vi "main.vi"() -> ()   [LabVIEW 2019]
uses:
  <vilib>/vision/Image Controls.llb/IMAQ Image.ctl
  <vilib>/Utility/error.llb/DialogType.ctl
  <vilib>/measure/mamon.llb/Trigger Detection for 1 Channel.vi
  <vilib>/vision/NI_Vision_Development_Module.lvlib
  <vilib>/measure/NI_MAPro.lvlib
panel:
  out "Frame Rate":dbl
  out "Speed.ER":bool
  out "error out 7":errorcluster
  out "error out 6":errorcluster
  out "error out 5":errorcluster
  out "pallet Movement (m)":dbl format="%.2g"
  out "Plt Count 2":bool
  out "pallet count accept":bool
  out "machine pallet speed":dbl format="%#_3g"
  out "Array 2":errorcluster[](array[cluster])
  in  "Login":bool=TRUE
  out "error out 3":errorcluster
  out "GB sit 2":i8
  out "DEF TYPE":string="1"
  out "Sen.ER":bool
  out "Cam.ER":bool
  out "tcp read stop":bool
  out "main loop stop":bool
  out "event loop stop":bool
  out "sensor loop stop":bool
  out "stop ok":bool caption="YES"
  out "error out 2":errorcluster
  out "capture or not? 2":bool=TRUE
  out "stop live view":bool
  out "camera error out":errorcluster
  out "camera error in":errorcluster
  out "snap img":T1
  out "error out":errorcluster
  out "Array":dbl[][](array[numeric])
  out "SW&col sit":T2
  out "curv Array out":dbl[](array[numeric])
  out "capture or not?":bool=TRUE
  in  "Button":bool
  out "Frm False":bool
  out "Run/Stop":bool
  out "Sync":bool
  out "Speed (m/min) :":string="0"
  out "PLT NUM :":string="1"
  out "time&date 2":string="08:00:00"
  out "time&date":string="2020/11/22"
  out "Plt Count":bool
  out "Col. Count":bool
  in  "Sequence Button":bool
  in  "setting":bool
  in  "Graph Button":bool
  in  "report":bool
  in  "stop 3":bool
  out "DPIS":string="DPIS"
  in  "capture":bool
  out "Sen Plt\nNUM":i16
  out "CURV (mm)":dbl format="%#.2g"
  out "GB defects%":dbl format="%#.1g"
  out "Alarm":bool
  in  "OFF":bool
  out "Pallet Defects View":T1(plugin-control)
  out "GB sit":u32(colorbox)=16448250
  out "curv sit":bool
  out "SWR 2":bool
  out "SWL 2":bool
  in  "Refresh Button":bool
  in  "PLT NUM SYNC":i16
  out "Col\n NUM":dbl format="%#.1g"
  out "Live View":T1(plugin-control)
  out "bottum loop stop":bool
  out "stop ok":bool caption="OK"
  out "bottum refrence":refnum<vi>[](array[refnum])
  out "bottum array":bool[](array[boolean])
  in  "232":bool
  in  "231":bool
  in  "230":bool
  in  "229":bool
  in  "228":bool
  in  "227":bool
  in  "226":bool
  in  "225":bool
  in  "224":bool
  in  "223":bool
  in  "222":bool
  in  "221":bool
  in  "220":bool
  in  "219":bool
  in  "218":bool
  in  "217":bool
  in  "216":bool
  in  "215":bool
  in  "214":bool
  in  "213":bool
  in  "212":bool
  in  "211":bool
  in  "210":bool
  in  "209":bool
  in  "208":bool
  in  "207":bool
  in  "206":bool
  in  "205":bool
  in  "204":bool
  in  "203":bool
  in  "202":bool
  in  "201":bool
  in  "200":bool
  in  "199":bool
  in  "198":bool
  in  "197":bool
  in  "196":bool
  in  "195":bool
  in  "194":bool
  in  "193":bool
  in  "192":bool
  in  "191":bool
  in  "190":bool
  in  "189":bool
  in  "188":bool
  in  "187":bool
  in  "186":bool
  in  "185":bool
  in  "184":bool
  in  "183":bool
  in  "182":bool
  in  "181":bool
  in  "180":bool
  in  "179":bool
  in  "178":bool
  in  "177":bool
  in  "176":bool
  in  "175":bool
  in  "174":bool
  in  "173":bool
  in  "172":bool
  in  "171":bool
  in  "170":bool
  in  "169":bool
  in  "168":bool
  in  "167":bool
  in  "166":bool
  in  "165":bool
  in  "164":bool
  in  "163":bool
  in  "162":bool
  in  "161":bool
  in  "160":bool
  in  "159":bool
  in  "158":bool
  in  "157":bool
  in  "156":bool
  in  "155":bool
  in  "154":bool
  in  "153":bool
  in  "152":bool
  in  "151":bool
  in  "150":bool
  in  "149":bool
  in  "148":bool
  in  "147":bool
  in  "146":bool
  in  "145":bool
  in  "144":bool
  in  "143":bool
  in  "142":bool
  in  "141":bool
  in  "140":bool
  in  "139":bool
  in  "138":bool
  in  "137":bool
  in  "136":bool
  in  "135":bool
  in  "134":bool
  in  "133":bool
  in  "132":bool
  in  "131":bool
  in  "130":bool
  in  "129":bool
  in  "128":bool
  in  "127":bool
  in  "126":bool
  in  "125":bool
  in  "124":bool
  in  "123":bool
  in  "122":bool
  in  "121":bool
  in  "120":bool
  in  "119":bool
  in  "118":bool
  in  "117":bool
  in  "1":bool
  in  "2":bool
  in  "3":bool
  in  "4":bool
  in  "5":bool
  in  "6":bool
  in  "7":bool
  in  "8":bool
  in  "9":bool
  in  "10":bool
  in  "11":bool
  in  "12":bool
  in  "13":bool
  in  "14":bool
  in  "15":bool
  in  "16":bool
  in  "17":bool
  in  "18":bool
  in  "19":bool
  in  "20":bool
  in  "21":bool
  in  "22":bool
  in  "23":bool
  in  "24":bool
  in  "25":bool
  in  "26":bool
  in  "27":bool
  in  "28":bool
  in  "29":bool
  in  "30":bool
  in  "31":bool
  in  "32":bool
  in  "33":bool
  in  "34":bool
  in  "35":bool
  in  "36":bool
  in  "37":bool
  in  "38":bool
  in  "39":bool
  in  "40":bool
  in  "41":bool
  in  "42":bool
  in  "43":bool
  in  "44":bool
  in  "45":bool
  in  "46":bool
  in  "47":bool
  in  "48":bool
  in  "49":bool
  in  "50":bool
  in  "51":bool
  in  "52":bool
  in  "53":bool
  in  "54":bool
  in  "55":bool
  in  "56":bool
  in  "57":bool
  in  "58":bool
  in  "59":bool
  in  "60":bool
  in  "61":bool
  in  "62":bool
  in  "63":bool
  in  "64":bool
  in  "65":bool
  in  "66":bool
  in  "67":bool
  in  "68":bool
  in  "69":bool
  in  "70":bool
  in  "71":bool
  in  "72":bool
  in  "73":bool
  in  "74":bool
  in  "75":bool
  in  "76":bool
  in  "77":bool
  in  "78":bool
  in  "79":bool
  in  "80":bool
  in  "81":bool
  in  "82":bool
  in  "83":bool
  in  "84":bool
  in  "85":bool
  in  "86":bool
  in  "87":bool
  in  "88":bool
  in  "89":bool
  in  "90":bool
  in  "91":bool
  in  "92":bool
  in  "93":bool
  in  "94":bool
  in  "95":bool
  in  "96":bool
  in  "97":bool
  in  "98":bool
  in  "99":bool
  in  "100":bool
  in  "101":bool
  in  "102":bool
  in  "103":bool
  in  "104":bool
  in  "105":bool
  in  "106":bool
  in  "107":bool
  in  "108":bool
  in  "109":bool
  in  "110":bool
  in  "111":bool
  in  "112":bool
  in  "113":bool
  in  "114":bool
  in  "115":bool
  in  "116":bool
types:
  T1 = typedef "IMAQ Image.ctl" = refnum<image>
  T2 = cluster{"curv sit":bool, "Right Sidewall":bool, "Left SideWall":bool}
  T3 = typedef "Image Type" = u32
  T4 = enum8{"Enabled", "Disabled", "Disabled and Grayed Out"}
  T5 = typedef "DialogType.ctl" = u16
  T6 = cluster{"plt number dis":i16, "Table Name":string, "Database Name":string, "DB days to save":i16, "IP #":string, "Img Path":path, "Port":u16, "time out":u16, "madule path":path, "IP # speed":string, "counting device":enum16{"Sensors", "Line Speed", "Sensors&Speed"}}
  T7 = cluster{"ch sensor1":dbl, "ch sensor2":dbl, "chs ensor3":dbl, "ch sw sensor1":dbl, "ch sw sensor2":dbl}
  T8 = cluster{"low level read thr 1":dbl, "low level read thr 2":dbl, "low level read thr 3":dbl, "Debounce Time":dbl, "falling level thr":dbl, "counting role 2":enum16{"1st sensor", "2nd sensor", "3rd sensor", "1st+2nd", "1st+3rd", "2nd+3rd", "1st+2nd+3rd"}}
  T9 = enum16{"1st sensor", "2nd sensor", "3rd sensor", "1st+2nd", "1st+3rd", "2nd+3rd", "1st+2nd+3rd"}
  T10 = cluster{"Curv thr (mm)":dbl, "SW timout(s)":dbl, "SWR thr":dbl, "SWL thr ":dbl}
  T11 = cluster{"curv sit":bool, "right SideWall ":bool, "Left SideWall":bool}
  T12 = cluster{"min box size":dbl, "max box size":dbl, "box ratio":dbl, "min area size(gap)":dbl, "max area size (gap)":dbl, "min area (hole)":dbl, "max area (hole)":dbl}
  T13 = enum32{"Invalid", "Standard", "Closed", "Hidden", "Minimized", "Maximized"}
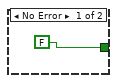
[diagram p3: hidden frame]
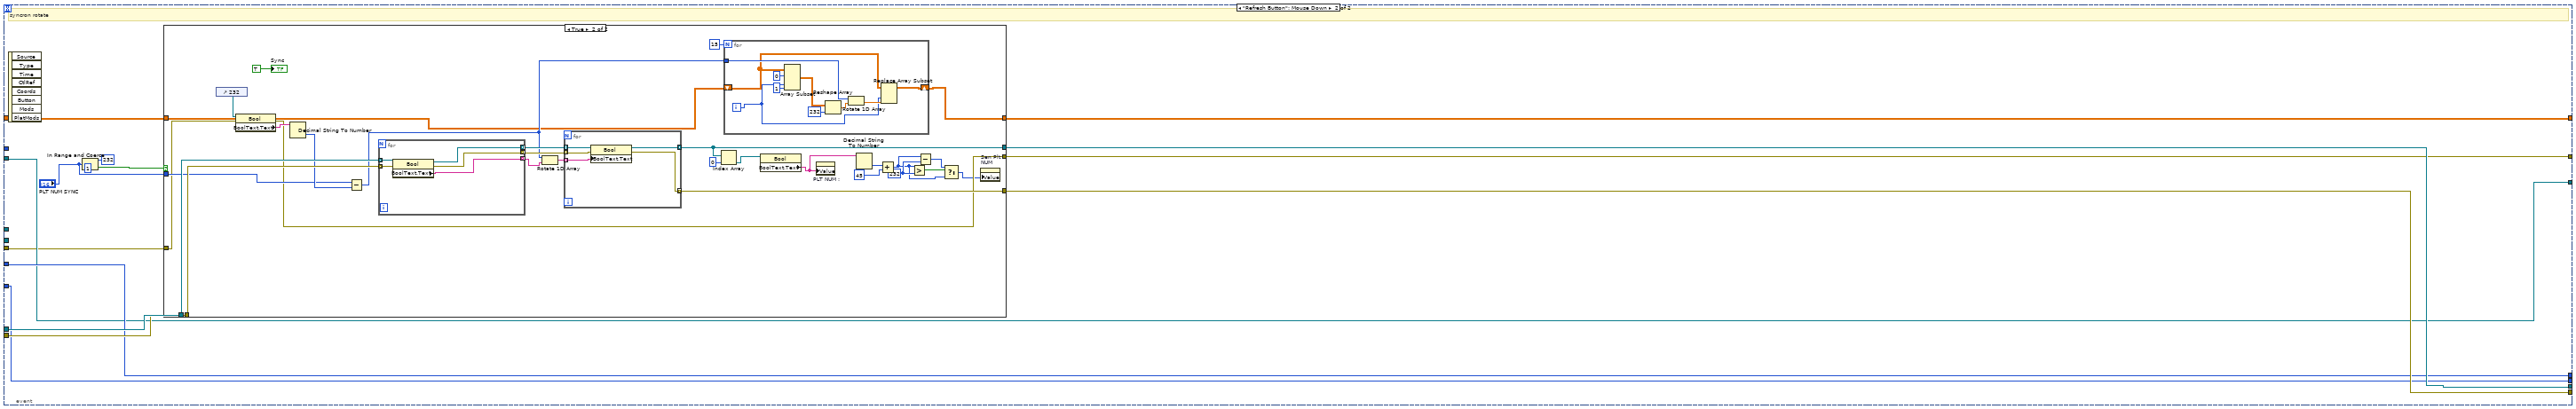
[diagram p6: hidden frame]
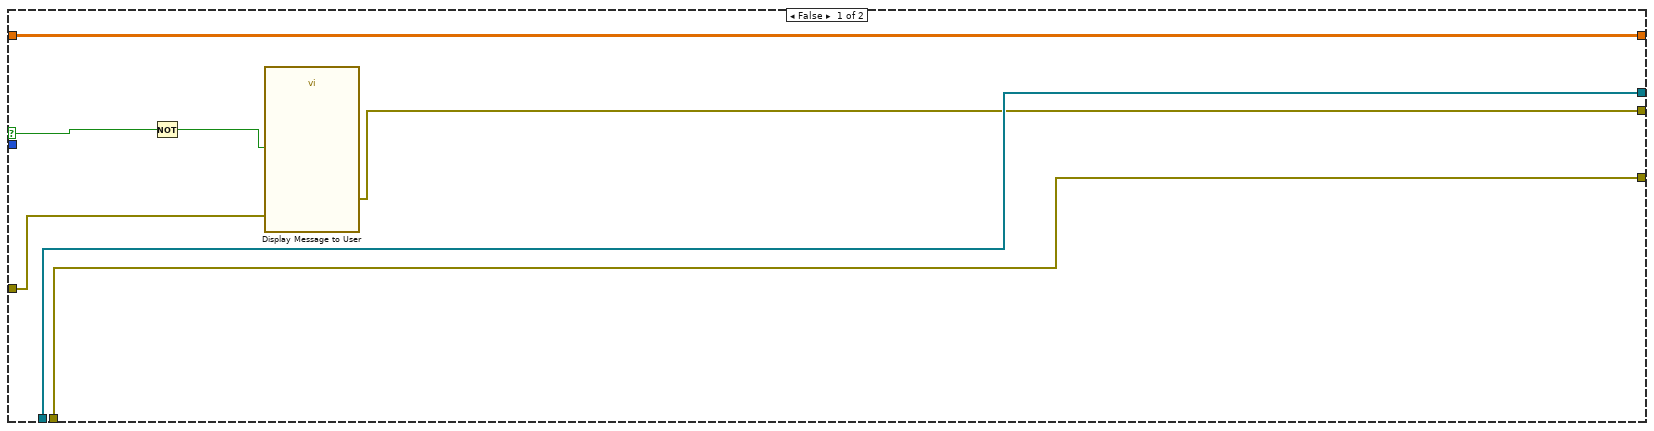
[diagram p7: hidden frame]
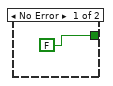
[diagram p8: hidden frame]
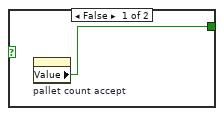
[diagram p10: hidden frame]
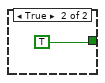
[diagram p11: hidden frame]
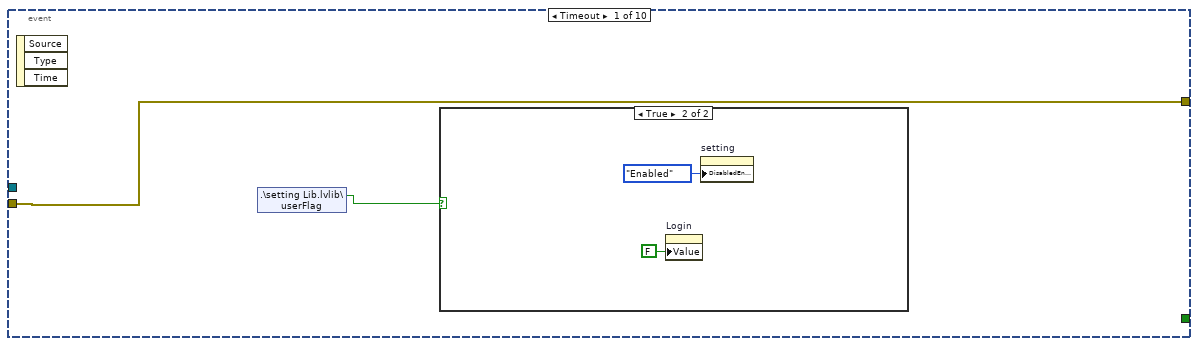
[diagram p12: hidden frame]
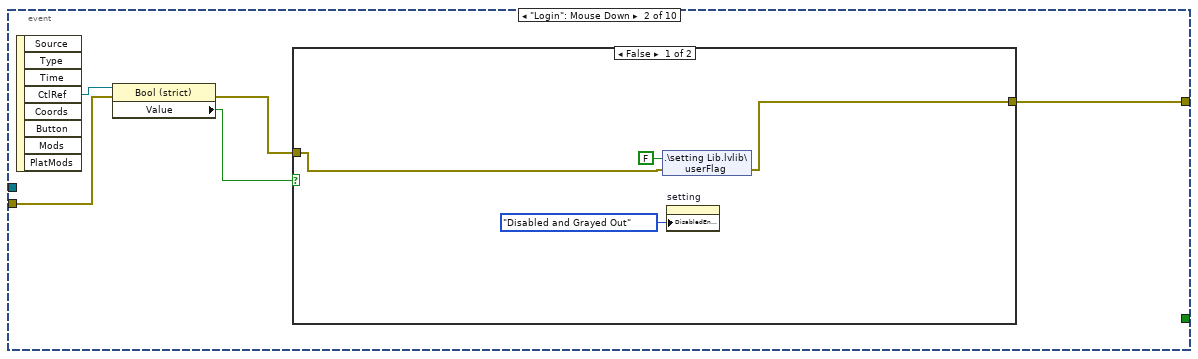
[diagram p14: hidden frame]
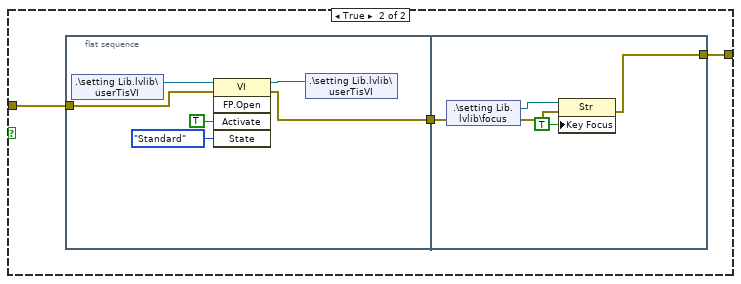
[diagram p15: hidden frame]
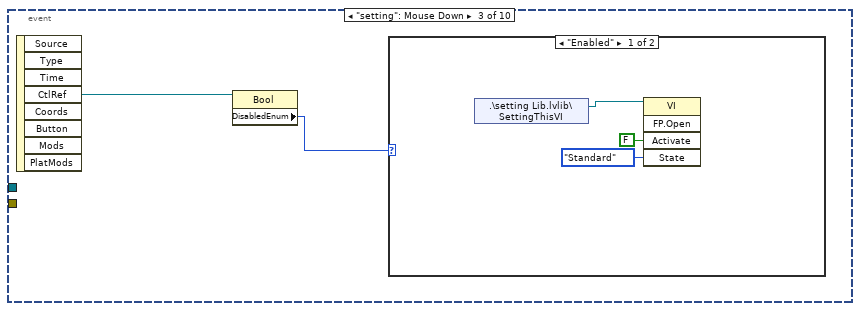
[diagram p16: hidden frame]
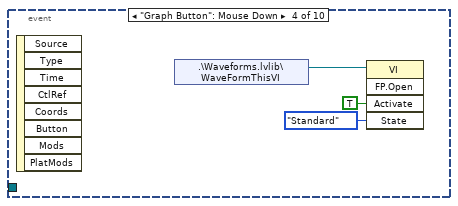
[diagram p18: hidden frame]
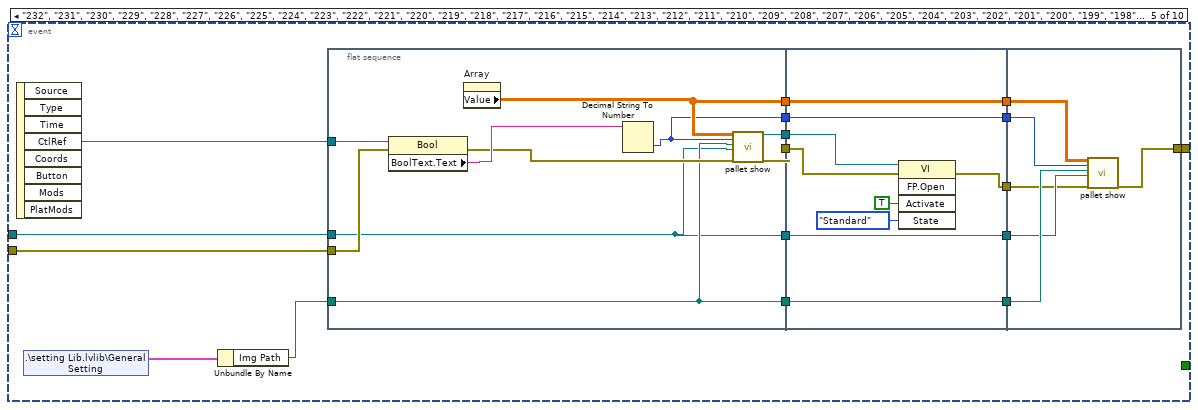
[diagram p19: hidden frame]
diagram:
  w2 = T3 0 items=["Grayscale (U8)", "Grayscale (I16)", "Grayscale (SGL)", "Complex (CSG)", "RGB (U32)", "HSL (U32)", "RGB (U64)", "Grayscale (U16)"] ("Image Type")
  w3 = T3 0 items=["Grayscale (U8)", "Grayscale (I16)", "Grayscale (SGL)", "Complex (CSG)", "RGB (U32)", "HSL (U32)", "RGB (U64)", "Grayscale (U16)"] ("Image Type")
  w32 = FALSE ("main loop stop")
  w40 = FALSE ("Plt Count")
  w59 = T3 4 items=["Grayscale (U8)", "Grayscale (I16)", "Grayscale (SGL)", "Complex (CSG)", "RGB (U32)", "HSL (U32)", "RGB (U64)", "Grayscale (U16)"] ("Image Type")
  w85 = 250 ("dimension size")
  w90 = 2 ("dimension size")
  w94 = 25 ("dimension size")
  n1 = while {
    tunnel: [w342] -> w109
    stop <- w342 stop-if-true
    n2 = Wait (ms)(milliseconds to wait=u32 5) -> ()  [unwired: 1 out]
    n3 = local read "stop ok"() -> (w342:bool)
    n4 = Build Array("232", "231", "230", "229", "228", "227", "226", "225", "224", "223", "222", "221", "220", "219", "218", "217", "216", "215", "214", "213", "212", "211", "210", "209", "208", "207", "206", "205", "204", "203", "202", "201", "200", "199", "198", "197", "196", "195", "194", "193", "192", "191", "190", "189", "188", "187", "186", "185", "184", "183", "182", "181", "180", "179", "178", "177", "176", "175", "174", "173", "172", "171", "170", "169", "168", "167", "166", "165", "164", "163", "162", "161", "160", "159", "158", "157", "156", "155", "154", "153", "152", "151", "150", "149", "148", "147", "146", "145", "144", "143", "142", "141", "140", "139", "138", "137", "136", "135", "134", "133", "132", "131", "130", "129", "128", "127", "126", "125", "124", "123", "122", "121", "120", "119", "118", "117", "116", "115", "114", "113", "112", "111", "110", "109", "108", "107", "106", "105", "104", "103", "102", "101", "100", "99", "98", "97", "96", "95", "94", "93", "92", "91", "90", "89", "88", "87", "86", "85", "84", "83", "82", "81", "80", "79", "78", "77", "76", "75", "74", "73", "72", "71", "70", "69", "68", "67", "66", "65", "64", "63", "62", "61", "60", "59", "58", "57", "56", "55", "54", "53", "52", "51", "50", "49", "48", "47", "46", "45", "44", "43", "42", "41", "40", "39", "38", "37", "36", "35", "34", "33", "32", "31", "30", "29", "28", "27", "26", "25", "24", "23", "22", "21", "20", "19", "18", "17", "16", "15", "14", "13", "12", "11", "10", "9", "8", "7", "6", "5", "4", "3", "2", "1") -> (→"bottum array":bool[])
  }
  "bottum loop stop" <- w109
  n5 = control-ref of="232"() -> (w341:refnum<vi>)
  n6 = control-ref of="231"() -> (w340:refnum<vi>)
  n7 = control-ref of="230"() -> (w339:refnum<vi>)
  n8 = control-ref of="229"() -> (w338:refnum<vi>)
  n9 = control-ref of="228"() -> (w337:refnum<vi>)
  n10 = control-ref of="227"() -> (w336:refnum<vi>)
  n11 = control-ref of="226"() -> (w335:refnum<vi>)
  n12 = control-ref of="225"() -> (w334:refnum<vi>)
  n13 = control-ref of="224"() -> (w333:refnum<vi>)
  n14 = control-ref of="223"() -> (w332:refnum<vi>)
  n15 = control-ref of="222"() -> (w331:refnum<vi>)
  n16 = control-ref of="221"() -> (w330:refnum<vi>)
  n17 = control-ref of="220"() -> (w329:refnum<vi>)
  n18 = control-ref of="219"() -> (w328:refnum<vi>)
  n19 = control-ref of="218"() -> (w327:refnum<vi>)
  n20 = control-ref of="217"() -> (w326:refnum<vi>)
  n21 = control-ref of="216"() -> (w325:refnum<vi>)
  n22 = control-ref of="215"() -> (w324:refnum<vi>)
  n23 = control-ref of="214"() -> (w323:refnum<vi>)
  n24 = control-ref of="213"() -> (w322:refnum<vi>)
  n25 = control-ref of="212"() -> (w321:refnum<vi>)
  n26 = control-ref of="211"() -> (w320:refnum<vi>)
  n27 = control-ref of="210"() -> (w319:refnum<vi>)
  n28 = control-ref of="209"() -> (w318:refnum<vi>)
  n29 = control-ref of="208"() -> (w317:refnum<vi>)
  n30 = control-ref of="207"() -> (w316:refnum<vi>)
  n31 = control-ref of="206"() -> (w315:refnum<vi>)
  n32 = control-ref of="205"() -> (w314:refnum<vi>)
  n33 = control-ref of="204"() -> (w313:refnum<vi>)
  n34 = control-ref of="203"() -> (w312:refnum<vi>)
  n35 = control-ref of="202"() -> (w311:refnum<vi>)
  n36 = control-ref of="201"() -> (w310:refnum<vi>)
  n37 = control-ref of="200"() -> (w309:refnum<vi>)
  n38 = control-ref of="199"() -> (w308:refnum<vi>)
  n39 = control-ref of="198"() -> (w307:refnum<vi>)
  n40 = control-ref of="197"() -> (w306:refnum<vi>)
  n41 = control-ref of="196"() -> (w305:refnum<vi>)
  n42 = control-ref of="195"() -> (w304:refnum<vi>)
  n43 = control-ref of="194"() -> (w303:refnum<vi>)
  n44 = control-ref of="193"() -> (w302:refnum<vi>)
  n45 = control-ref of="192"() -> (w301:refnum<vi>)
  n46 = control-ref of="191"() -> (w300:refnum<vi>)
  n47 = control-ref of="190"() -> (w299:refnum<vi>)
  n48 = control-ref of="189"() -> (w298:refnum<vi>)
  n49 = control-ref of="188"() -> (w297:refnum<vi>)
  n50 = control-ref of="187"() -> (w296:refnum<vi>)
  n51 = control-ref of="186"() -> (w295:refnum<vi>)
  n52 = control-ref of="185"() -> (w294:refnum<vi>)
  n53 = control-ref of="184"() -> (w293:refnum<vi>)
  n54 = control-ref of="183"() -> (w292:refnum<vi>)
  n55 = control-ref of="182"() -> (w291:refnum<vi>)
  n56 = control-ref of="181"() -> (w290:refnum<vi>)
  n57 = control-ref of="180"() -> (w289:refnum<vi>)
  n58 = control-ref of="179"() -> (w288:refnum<vi>)
  n59 = control-ref of="178"() -> (w287:refnum<vi>)
  n60 = control-ref of="177"() -> (w286:refnum<vi>)
  n61 = control-ref of="176"() -> (w285:refnum<vi>)
  n62 = control-ref of="175"() -> (w284:refnum<vi>)
  n63 = control-ref of="174"() -> (w283:refnum<vi>)
  n64 = control-ref of="173"() -> (w282:refnum<vi>)
  n65 = control-ref of="172"() -> (w281:refnum<vi>)
  n66 = control-ref of="171"() -> (w280:refnum<vi>)
  n67 = control-ref of="170"() -> (w279:refnum<vi>)
  n68 = control-ref of="169"() -> (w278:refnum<vi>)
  n69 = control-ref of="168"() -> (w277:refnum<vi>)
  n70 = control-ref of="167"() -> (w276:refnum<vi>)
  n71 = control-ref of="166"() -> (w275:refnum<vi>)
  n72 = control-ref of="165"() -> (w274:refnum<vi>)
  n73 = control-ref of="164"() -> (w273:refnum<vi>)
  n74 = control-ref of="163"() -> (w272:refnum<vi>)
  n75 = control-ref of="162"() -> (w271:refnum<vi>)
  n76 = control-ref of="161"() -> (w270:refnum<vi>)
  n77 = control-ref of="160"() -> (w269:refnum<vi>)
  n78 = control-ref of="159"() -> (w268:refnum<vi>)
  n79 = control-ref of="158"() -> (w267:refnum<vi>)
  n80 = control-ref of="157"() -> (w266:refnum<vi>)
  n81 = control-ref of="156"() -> (w265:refnum<vi>)
  n82 = control-ref of="155"() -> (w264:refnum<vi>)
  n83 = control-ref of="154"() -> (w263:refnum<vi>)
  n84 = control-ref of="153"() -> (w262:refnum<vi>)
  n85 = control-ref of="152"() -> (w261:refnum<vi>)
  n86 = control-ref of="151"() -> (w260:refnum<vi>)
  n87 = control-ref of="150"() -> (w259:refnum<vi>)
  n88 = control-ref of="149"() -> (w258:refnum<vi>)
  n89 = control-ref of="148"() -> (w257:refnum<vi>)
  n90 = control-ref of="147"() -> (w256:refnum<vi>)
  n91 = control-ref of="146"() -> (w255:refnum<vi>)
  n92 = control-ref of="145"() -> (w254:refnum<vi>)
  n93 = control-ref of="144"() -> (w253:refnum<vi>)
  n94 = control-ref of="143"() -> (w252:refnum<vi>)
  n95 = control-ref of="142"() -> (w251:refnum<vi>)
  n96 = control-ref of="141"() -> (w250:refnum<vi>)
  n97 = control-ref of="140"() -> (w249:refnum<vi>)
  n98 = control-ref of="139"() -> (w248:refnum<vi>)
  n99 = control-ref of="138"() -> (w247:refnum<vi>)
  n100 = control-ref of="137"() -> (w246:refnum<vi>)
  n101 = control-ref of="136"() -> (w245:refnum<vi>)
  n102 = control-ref of="135"() -> (w244:refnum<vi>)
  n103 = control-ref of="134"() -> (w243:refnum<vi>)
  n104 = control-ref of="133"() -> (w242:refnum<vi>)
  n105 = control-ref of="132"() -> (w241:refnum<vi>)
  n106 = control-ref of="131"() -> (w240:refnum<vi>)
  n107 = control-ref of="130"() -> (w239:refnum<vi>)
  n108 = control-ref of="129"() -> (w238:refnum<vi>)
  n109 = control-ref of="128"() -> (w237:refnum<vi>)
  n110 = control-ref of="127"() -> (w236:refnum<vi>)
  n111 = control-ref of="126"() -> (w235:refnum<vi>)
  n112 = control-ref of="125"() -> (w234:refnum<vi>)
  n113 = control-ref of="124"() -> (w233:refnum<vi>)
  n114 = control-ref of="123"() -> (w232:refnum<vi>)
  n115 = control-ref of="122"() -> (w231:refnum<vi>)
  n116 = control-ref of="121"() -> (w230:refnum<vi>)
  n117 = control-ref of="120"() -> (w229:refnum<vi>)
  n118 = control-ref of="119"() -> (w228:refnum<vi>)
  n119 = control-ref of="118"() -> (w227:refnum<vi>)
  n120 = control-ref of="117"() -> (w226:refnum<vi>)
  n121 = control-ref of="116"() -> (w225:refnum<vi>)
  n122 = control-ref of="115"() -> (w224:refnum<vi>)
  n123 = control-ref of="114"() -> (w223:refnum<vi>)
  n124 = control-ref of="113"() -> (w222:refnum<vi>)
  n125 = control-ref of="112"() -> (w221:refnum<vi>)
  n126 = control-ref of="111"() -> (w220:refnum<vi>)
  n127 = control-ref of="110"() -> (w219:refnum<vi>)
  n128 = control-ref of="109"() -> (w218:refnum<vi>)
  n129 = control-ref of="108"() -> (w217:refnum<vi>)
  n130 = control-ref of="107"() -> (w216:refnum<vi>)
  n131 = control-ref of="106"() -> (w215:refnum<vi>)
  n132 = control-ref of="105"() -> (w214:refnum<vi>)
  n133 = control-ref of="104"() -> (w213:refnum<vi>)
  n134 = control-ref of="103"() -> (w212:refnum<vi>)
  n135 = control-ref of="102"() -> (w211:refnum<vi>)
  n136 = control-ref of="101"() -> (w210:refnum<vi>)
  n137 = control-ref of="100"() -> (w209:refnum<vi>)
  n138 = control-ref of="99"() -> (w208:refnum<vi>)
  n139 = control-ref of="98"() -> (w207:refnum<vi>)
  n140 = control-ref of="97"() -> (w206:refnum<vi>)
  n141 = control-ref of="96"() -> (w205:refnum<vi>)
  n142 = control-ref of="95"() -> (w204:refnum<vi>)
  n143 = control-ref of="94"() -> (w203:refnum<vi>)
  n144 = control-ref of="93"() -> (w202:refnum<vi>)
  n145 = control-ref of="92"() -> (w201:refnum<vi>)
  n146 = control-ref of="91"() -> (w200:refnum<vi>)
  n147 = control-ref of="90"() -> (w199:refnum<vi>)
  n148 = control-ref of="89"() -> (w198:refnum<vi>)
  n149 = control-ref of="88"() -> (w197:refnum<vi>)
  n150 = control-ref of="87"() -> (w196:refnum<vi>)
  n151 = control-ref of="86"() -> (w195:refnum<vi>)
  n152 = control-ref of="85"() -> (w194:refnum<vi>)
  n153 = control-ref of="84"() -> (w193:refnum<vi>)
  n154 = control-ref of="83"() -> (w192:refnum<vi>)
  n155 = control-ref of="82"() -> (w191:refnum<vi>)
  n156 = control-ref of="81"() -> (w190:refnum<vi>)
  n157 = control-ref of="80"() -> (w189:refnum<vi>)
  n158 = control-ref of="79"() -> (w188:refnum<vi>)
  n159 = control-ref of="78"() -> (w187:refnum<vi>)
  n160 = control-ref of="77"() -> (w186:refnum<vi>)
  n161 = control-ref of="76"() -> (w185:refnum<vi>)
  n162 = control-ref of="75"() -> (w184:refnum<vi>)
  n163 = control-ref of="74"() -> (w183:refnum<vi>)
  n164 = control-ref of="73"() -> (w182:refnum<vi>)
  n165 = control-ref of="72"() -> (w181:refnum<vi>)
  n166 = control-ref of="71"() -> (w180:refnum<vi>)
  n167 = control-ref of="70"() -> (w179:refnum<vi>)
  n168 = control-ref of="69"() -> (w178:refnum<vi>)
  n169 = control-ref of="68"() -> (w177:refnum<vi>)
  n170 = control-ref of="67"() -> (w176:refnum<vi>)
  n171 = control-ref of="66"() -> (w175:refnum<vi>)
  n172 = control-ref of="65"() -> (w174:refnum<vi>)
  n173 = control-ref of="64"() -> (w173:refnum<vi>)
  n174 = control-ref of="63"() -> (w172:refnum<vi>)
  n175 = control-ref of="62"() -> (w171:refnum<vi>)
  n176 = control-ref of="61"() -> (w170:refnum<vi>)
  n177 = control-ref of="60"() -> (w169:refnum<vi>)
  n178 = control-ref of="59"() -> (w168:refnum<vi>)
  n179 = control-ref of="58"() -> (w167:refnum<vi>)
  n180 = control-ref of="57"() -> (w166:refnum<vi>)
  n181 = control-ref of="56"() -> (w165:refnum<vi>)
  n182 = control-ref of="55"() -> (w164:refnum<vi>)
  n183 = control-ref of="54"() -> (w163:refnum<vi>)
  n184 = control-ref of="53"() -> (w162:refnum<vi>)
  n185 = control-ref of="52"() -> (w161:refnum<vi>)
  n186 = control-ref of="51"() -> (w160:refnum<vi>)
  n187 = control-ref of="50"() -> (w159:refnum<vi>)
  n188 = control-ref of="49"() -> (w158:refnum<vi>)
  n189 = control-ref of="48"() -> (w157:refnum<vi>)
  n190 = control-ref of="47"() -> (w156:refnum<vi>)
  n191 = control-ref of="46"() -> (w155:refnum<vi>)
  n192 = control-ref of="45"() -> (w154:refnum<vi>)
  n193 = control-ref of="44"() -> (w153:refnum<vi>)
  n194 = control-ref of="43"() -> (w152:refnum<vi>)
  n195 = control-ref of="42"() -> (w151:refnum<vi>)
  n196 = control-ref of="41"() -> (w150:refnum<vi>)
  n197 = control-ref of="40"() -> (w149:refnum<vi>)
  n198 = control-ref of="39"() -> (w148:refnum<vi>)
  n199 = control-ref of="38"() -> (w147:refnum<vi>)
  n200 = control-ref of="37"() -> (w146:refnum<vi>)
  n201 = control-ref of="36"() -> (w145:refnum<vi>)
  n202 = control-ref of="35"() -> (w144:refnum<vi>)
  n203 = control-ref of="34"() -> (w143:refnum<vi>)
  n204 = control-ref of="33"() -> (w142:refnum<vi>)
  n205 = control-ref of="32"() -> (w141:refnum<vi>)
  n206 = control-ref of="31"() -> (w140:refnum<vi>)
  n207 = control-ref of="30"() -> (w139:refnum<vi>)
  n208 = control-ref of="29"() -> (w138:refnum<vi>)
  n209 = control-ref of="28"() -> (w137:refnum<vi>)
  n210 = control-ref of="27"() -> (w136:refnum<vi>)
  n211 = control-ref of="26"() -> (w135:refnum<vi>)
  n212 = control-ref of="25"() -> (w134:refnum<vi>)
  n213 = control-ref of="24"() -> (w133:refnum<vi>)
  n214 = control-ref of="23"() -> (w132:refnum<vi>)
  n215 = control-ref of="22"() -> (w131:refnum<vi>)
  n216 = control-ref of="21"() -> (w130:refnum<vi>)
  n217 = control-ref of="20"() -> (w129:refnum<vi>)
  n218 = control-ref of="19"() -> (w128:refnum<vi>)
  n219 = control-ref of="18"() -> (w127:refnum<vi>)
  n220 = control-ref of="17"() -> (w126:refnum<vi>)
  n221 = control-ref of="16"() -> (w125:refnum<vi>)
  n222 = control-ref of="15"() -> (w124:refnum<vi>)
  n223 = control-ref of="14"() -> (w123:refnum<vi>)
  n224 = control-ref of="13"() -> (w122:refnum<vi>)
  n225 = control-ref of="12"() -> (w121:refnum<vi>)
  n226 = control-ref of="11"() -> (w120:refnum<vi>)
  n227 = control-ref of="10"() -> (w119:refnum<vi>)
  n228 = control-ref of="9"() -> (w118:refnum<vi>)
  n229 = control-ref of="8"() -> (w117:refnum<vi>)
  n230 = control-ref of="7"() -> (w116:refnum<vi>)
  n231 = control-ref of="6"() -> (w115:refnum<vi>)
  n232 = control-ref of="5"() -> (w114:refnum<vi>)
  n233 = control-ref of="4"() -> (w113:refnum<vi>)
  n234 = control-ref of="3"() -> (w112:refnum<vi>)
  n235 = control-ref of="2"() -> (w111:refnum<vi>)
  n236 = control-ref of="1"() -> (w110:refnum<vi>)
  n237 = property on="Run/Stop" class="Bool (strict)"("Blinking"=FALSE) -> ()  [unwired: 2 in, 2 out]
  n238 = property on="Alarm" class="Bool (strict)"("Blinking"=FALSE) -> ()  [unwired: 2 in, 2 out]
  n239 = property on="Sync" class="Bool (strict)"("Value"=FALSE ("Sync")) -> ()  [unwired: 2 in, 2 out]
  n240 = property on="Run/Stop" class="Bool (strict)"("Value"=TRUE ("Run/Stop")) -> ()  [unwired: 2 in, 2 out]
  n241 = property on="event loop stop" class="Bool (strict)"("Value"=w32) -> ()  [unwired: 2 in, 2 out]
  n242 = property on="tcp read stop" class="Bool (strict)"("Value"=w32) -> ()  [unwired: 2 in, 2 out]
  n243 = property on="stop live view" class="Bool (strict)"("Value"=w32) -> ()  [unwired: 2 in, 2 out]
  n244 = property on="sensor loop stop" class="Bool (strict)"("Value"=w32) -> ()  [unwired: 2 in, 2 out]
  n245 = property on="main loop stop" class="Bool (strict)"("Value"=w32) -> ()  [unwired: 2 in, 2 out]
  n246 = property on="Col\n NUM" class="DigNum (strict)"("Value"=0.0 ("Col\n NUM")) -> ()  [unwired: 2 in, 2 out]
  n247 = property on="Sen Plt\nNUM" class="DigNum (strict)"("Value"=i16 46 ("Sen Plt\nNUM")) -> ()  [unwired: 2 in, 2 out]
  n248 = property on="PLT NUM SYNC" class="DigNum (strict)"("Value"=i16 1 ("PLT NUM SYNC")) -> ()  [unwired: 2 in, 2 out]
  n249 = property on="CURV (mm)" class="DigNum (strict)"("Value"=0.0 ("CURV (mm)")) -> ()  [unwired: 2 in, 2 out]
  n250 = property on="GB defects%" class="DigNum (strict)"("Value"=0.0 ("GB defects%")) -> ()  [unwired: 2 in, 2 out]
  n251 = property on="PLT NUM :" class="Str"("Value"="1" ("PLT NUM :")) -> ()  [unwired: 2 in, 2 out]
  n252 = Build Array(w341, w340, w339, w338, w337, w336, w335, w334, w333, w332, w331, w330, w329, w328, w327, w326, w325, w324, w323, w322, w321, w320, w319, w318, w317, w316, w315, w314, w313, w312, w311, w310, w309, w308, w307, w306, w305, w304, w303, w302, w301, w300, w299, w298, w297, w296, w295, w294, w293, w292, w291, w290, w289, w288, w287, w286, w285, w284, w283, w282, w281, w280, w279, w278, w277, w276, w275, w274, w273, w272, w271, w270, w269, w268, w267, w266, w265, w264, w263, w262, w261, w260, w259, w258, w257, w256, w255, w254, w253, w252, w251, w250, w249, w248, w247, w246, w245, w244, w243, w242, w241, w240, w239, w238, w237, w236, w235, w234, w233, w232, w231, w230, w229, w228, w227, w226, w225, w224, w223, w222, w221, w220, w219, w218, w217, w216, w215, w214, w213, w212, w211, w210, w209, w208, w207, w206, w205, w204, w203, w202, w201, w200, w199, w198, w197, w196, w195, w194, w193, w192, w191, w190, w189, w188, w187, w186, w185, w184, w183, w182, w181, w180, w179, w178, w177, w176, w175, w174, w173, w172, w171, w170, w169, w168, w167, w166, w165, w164, w163, w162, w161, w160, w159, w158, w157, w156, w155, w154, w153, w152, w151, w150, w149, w148, w147, w146, w145, w144, w143, w142, w141, w140, w139, w138, w137, w136, w135, w134, w133, w132, w131, w130, w129, w128, w127, w126, w125, w124, w123, w122, w121, w120, w119, w118, w117, w116, w115, w114, w113, w112, w111, w110) -> (w108:refnum<vi>[])
  "bottum refrence" <- w108
  n253 = while {
    tunnel: errorcluster {"status"=FALSE, "code"=0, "source"=""} ("error in (no error)") -> [w589]
    tunnel: [w585] -> w99
    tunnel: [w584] -> w98
    tunnel: [w577] -> w33
    stop <- w577 stop-if-true
    w586 = T5 0 items=["no dialog", "OK message", "continue or stop message", "OK message + warnings", "continue/stop + warnings"] ("type of dialog (OK msg:1)")
    n254 = shared-variable ".\\setting Lib.lvlib\\General Setting"() -> (w583:T6)  [unwired: 1 in, 1 out]
    n255 = Unbundle By Name(w583) -> ("IP #"=w582:string, "Port"=w581:u16)
    n256 = TCP Open Connection(address=w582, remote port or service name=w581, timeout ms (60000)=-1, error in (no error)=w589) -> (connection ID=w585:refnum<k5>, error out=w588:errorcluster)  [unwired: 1 in]
    n257 = shared-variable ".\\setting Lib.lvlib\\StopOk"() -> (w579:bool)  [unwired: 1 in, 1 out]
    n258 = call <vilib>:"Simple Error Handler.vi"("type of dialog (OK msg:1)"=w586, "error in (no error)"=w588) -> ("error?"=w587:bool, "error out"=w584:errorcluster)  [unwired: 3 in, 3 out]
    n259 = Not(x=w587) -> (.not. x?=w578:bool)
    n260 = Wait (ms)(milliseconds to wait=u32 5) -> ()  [unwired: 1 out]
    n261 = Or(x=w579, y=w578) -> (x .or. y?=w577:bool)
  }
  "tcp read stop" <- w33
  n262 = while {
    tunnel: errorcluster {"status"=FALSE, "code"=0, "source"=""} ("error in (no error)") -> [w603]
    tunnel: [w599] -> w19
    tunnel: [w598] -> w18
    tunnel: [w592] -> _
    stop <- w592 stop-if-true
    w600 = T5 0 items=["no dialog", "OK message", "continue or stop message", "OK message + warnings", "continue/stop + warnings"] ("type of dialog (OK msg:1)")
    n263 = shared-variable ".\\setting Lib.lvlib\\General Setting"() -> (w597:T6)  [unwired: 1 in, 1 out]
    n264 = Unbundle By Name(w597) -> ("IP # speed"=w596:string, "Port"=w591:u16)
    n265 = TCP Open Connection(address=w596, remote port or service name=w591, timeout ms (60000)=-1, error in (no error)=w603) -> (connection ID=w599:refnum<k5>, error out=w602:errorcluster)  [unwired: 1 in]
    n266 = shared-variable ".\\setting Lib.lvlib\\StopOk"() -> (w594:bool)  [unwired: 1 in, 1 out]
    n267 = call <vilib>:"Simple Error Handler.vi"("type of dialog (OK msg:1)"=w600, "error in (no error)"=w602) -> ("error?"=w601:bool, "error out"=w598:errorcluster)  [unwired: 3 in, 3 out]
    n268 = Not(x=w601) -> (.not. x?=w593:bool)
    n269 = Wait (ms)(milliseconds to wait=u32 5) -> ()  [unwired: 1 out]
    n270 = Or(x=w594, y=w593) -> (x .or. y?=w592:bool)
  }
  n271 = call "IMAQ Create"("Image Name"="mainimg", "Image Type"=w3, "error in (no error)"=errorcluster {"status"=FALSE, "code"=0, "source"=""}) -> ("New Image"=w56:T1, "error out"=w4:errorcluster)  [unwired: 2 in]
  n272 = control-ref of="Button"() -> (w107:refnum<vi>)
  n273 = property class="Bool"(reference=w107) -> ("Colors [4]"=w106:cluster{u32, u32}[])  [unwired: 1 in, 2 out]
  n274 = Initialize Array(i16 0 ("element"), 232 ("dimension size")) -> (w103:i16[])
  n275 = call "IMAQ Create"("Image Name"="rotate", "Image Type"=w2, "error in (no error)"=w4) -> ("New Image"=w49:T1, "error out"=w1:errorcluster)  [unwired: 2 in]
  n276 = for {
    tunnel: w108 -> [w617] mode=indexing
    tunnel: w106 -> [w612]
    shift-right: [w607] -> _
    shift-left: w103 -> [w609]
    tunnel: [w606] -> w102 mode=indexing
    tunnel: [w605] -> w101 mode=indexing
    i -> [w608]
    # "initialize text and label and colour of pallets"
    n277 = property class="Bool"(reference=w617) -> (reference out=w616:refnum<vi>, error out=w614:errorcluster, "Label.Text"=w615:string)  [unwired: 1 in]
    n278 = Replace Array Subset(array=w609, new element=w608, index=w608) -> (w607:i16[])
    n279 = property class="Bool"(reference=w616, error in=w614, "BoolText.Text"=w615) -> (reference out=w613:refnum<vi>)  [unwired: 1 out]
    n280 = property class="Bool"(reference=w613, "Colors [4]"=w612) -> (reference out=w611:refnum<vi>)  [unwired: 1 in, 1 out]
    n281 = property class="Bool"(reference=w611, "DisabledEnum"=T4."Disabled and Grayed Out" ("Disabled")) -> (reference out=w606:refnum<vi>, error out=w605:errorcluster)  [unwired: 1 in]
  }
  n282 = property on="capture or not?" class="Bool (strict)"("Value"=FALSE ("capture")) -> ()  [unwired: 2 in, 2 out]
  n283 = Open Python Session(python version="3.6" ("Python version"), 3:errorcluster {"status"=FALSE, "code"=0, "source"=""} ("error in (no error)")) -> (session out=w77:refnum<k35>, error out=w43:errorcluster)  [unwired: 1 in]
  n284 = while {
    tunnel: w56 -> [w638]
    tunnel: [w626] -> w53
    tunnel: [w630] -> w51
    tunnel: w49 -> [w639]
    tunnel: [w622] -> w48
    tunnel: w1 -> [w618]
    stop <- w626 stop-if-true
    # "Live view"
    n285 = flat-sequence {
      tunnel: w638 -> [w642]
      tunnel: w639 -> [w643]
      tunnel: [w643] -> w621
      tunnel: [w642] -> w620
      tunnel: [w641] -> w619
      tunnel: w618 -> [w641]
      tunnel: [w646] -> w637
      tunnel: [w644] -> w636
      tunnel: [w648] -> w635
      tunnel: [w647] -> w634
      tunnel: w621 -> [w648]
      tunnel: w620 -> [w647]
      tunnel: w619 -> [_]
      tunnel: w637 -> [w649]
      tunnel: w636 -> [w651]
      tunnel: w635 -> [w655]
      tunnel: w634 -> [w652]
      tunnel: [w655] -> w633
      tunnel: [w654] -> w632
      tunnel: [w650] -> w631
      tunnel: [w650] -> w627
      tunnel: w633 -> [w658]
      tunnel: w632 -> [w660]
      tunnel: w631 -> [w659]
      tunnel: [w661] -> w629
      tunnel: [w657] -> w628
      tunnel: w627 -> [w656]
      tunnel: [w662] -> w630
      tunnel: [w663] -> w622
      tunnel: w628 -> [w662]
      tunnel: w629 -> [w663]
      frame #0 {
      }
      frame #1 {
        (unwired) 10000 ("Timeout (ms)")
        n286 = call "Vision Acquisition"() -> ("Image Out"=w644:T1, "Frame Rate"=→"Frame Rate":dbl, "error out"=w646:errorcluster)  [unwired: 24 in, 1 out]
      }
      frame #2 {
        n287 = call "IMAQ Rotate"("error in (no error)"=w649, "Angle (degrees)"=sgl 180.0, "Image Dst"=w652, "Image Src"=w651) -> ("error out"=w654:errorcluster, "Image Dst Out"=w650:T1)  [unwired: 6 in]
      }
      frame #3 {
        n288 = call "IMAQ Copy"("error in (no error)"=w660, "Image Dst"=w658, "Image Src"=w659) -> ("error out"=w661:errorcluster, "Image Dst Out"=w657:T1)  [unwired: 3 in]
        "Live View" <- w656
      }
      frame #4 {
        "snap img" <- w662
      }
    }
    n289 = Wait (ms)(milliseconds to wait=u32 20) -> ()  [unwired: 1 out]
    n290 = shared-variable ".\\setting Lib.lvlib\\StopOk"() -> (w626:bool)  [unwired: 1 in, 1 out]
    n291 = Select(t=TRUE, s=w622, f=FALSE) -> (s? t:f=→"Cam.ER":bool)
    "camera error in" <- w622
  }
  "stop live view" <- w53
  n292 = Initialize Array(0.0 ("element"), w90, 2 ("dimension size")) -> (w91:dbl[][])
  n293 = Initialize Array(0.0 ("element"), w94, 3 ("dimension size")) -> (w95:dbl[][])
  n294 = property on="Col. Count" class="Bool (strict)"("Value"=FALSE ("Col. Count")) -> ()  [unwired: 2 in, 2 out]
  n295 = shared-variable ".\\setting Lib.lvlib\\StopOk"(FALSE ("StopOk")) -> ()  [unwired: 1 in, 1 out]
  n296 = call "IMAQ Create"("Image Name"="img crop", "error in (no error)"=w43) -> ("New Image"=w73:T1, "error out"=w74:errorcluster)  [unwired: 3 in]
  n297 = Initialize Array(0.0 ("element"), 6 ("dimension size")) -> (w81:dbl[])
  n298 = Initialize Array(0.0 ("element"), w85, 3 ("dimension size")) -> (w86:dbl[][])
  n299 = while {
    tunnel: w19 -> [w681]
    tunnel: w18 -> [w680]
    tunnel: [w669] -> w13
    stop <- FALSE stop-if-true
    n300 = call "adamread.vi"("TCP Connection Refnum in"=w681, "error in (no error)"=w680) -> ("Slave Input Registers 2"=w679:dbl[], "error out 2"=w669:errorcluster)  [unwired: 11 in, 1 out]
    n301 = Index Array(array=w679, index=3) -> (element=w677:dbl)
    n302 = Multiply(x=w677, y=0.000129) -> (x*y=w665:dbl)
    n303 = Greater?(x=w665, y=3.5) -> (0:w667:bool)
    n304 = case shown="False" w667 {
      tunnel: w665 -> [w683 w685]
      tunnel: [w684 w685] -> w664
      frame False {
        n305 = Multiply(x=w683, y=1.04) -> (x*y=w684:dbl)
      }
      frame True {
      }
    }
    "machine pallet speed" <- w664
    n306 = Number To Fractional String(number=w664, precision (6)=i16 2 ("width (-)")) -> (F-format string=→"Speed (m/min) :":string)  [unwired: 2 in]
    n307 = Greater?(x=w664, y=0.5) -> (0:→"Run/Stop":bool)
    n308 = case shown="Error .." w669 {
      tunnel: [FALSE ("Speed.ER") TRUE ("Speed.ER")] -> w668
      frame No Error {
      }
      frame Error {
      }
    }
    "Speed.ER" <- w668
    n309 = Wait (ms)(milliseconds to wait=u32 2000) -> ()  [unwired: 1 out]
  }
  "error out 7" <- w13
  n310 = Initialize Array(u32 0 ("element"), 400 ("dimension size"), 4 ("dimension size")) -> (w67:u32[][])
  n311 = Initialize Array "Crv&Sw info"(0.0 ("element"), 232 ("dimension size"), 16 ("dimension size")) -> (w63:dbl[][])
  n312 = call "IMAQ Create"("Image Name"="img out", "error in (no error)"=w74) -> ("New Image"=w72:T1, "error out"=w75:errorcluster)  [unwired: 3 in]
  n313 = call "defects database show.vi"() -> ()  [unwired: 12 in]
  n314 = call "query 2.vi"() -> ()  [unwired: 27 in, 1 out]
  n315 = Initialize Array(0.0 ("element"), 2 ("dimension size")) -> (w6:dbl[])
  n316 = Initialize Array(0.0 ("element"), 2 ("dimension size")) -> (w15:dbl[])
  n317 = property on="setting" class="Bool"("DisabledEnum"=T4."Disabled and Grayed Out" ("Disabled")) -> ()  [unwired: 2 in, 2 out]
  n318 = property on="capture or not? 2" class="Bool (strict)"("Value"=FALSE ("capture or not? 2")) -> ()  [unwired: 2 in, 2 out]
  n319 = call "user login.vi"() -> ()  [unwired: 12 in]
  n320 = property on="Plt Count" class="Bool (strict)"("Value"=w40) -> ()  [unwired: 2 in, 2 out]
  n321 = property on="Col. Count" class="Bool (strict)"("Value"=w40) -> ()  [unwired: 2 in, 2 out]
  n322 = call "setting page 2.vi"() -> ()  [unwired: 15 in, 1 out]
  n323 = call "IMAQ Create"("Image Name"="pallet show", "Image Type"=w59, "error in (no error)"=errorcluster {"status"=FALSE, "code"=0, "source"=""}) -> ("New Image"=w60:T1, "error out"=w42:errorcluster)  [unwired: 2 in]
  n324 = shared-variable ".\\setting Lib.lvlib\\userFlag"(FALSE ("userFlag")) -> ()  [unwired: 1 in, 1 out]
  n325 = property on="Login" class="Bool (strict)"("Value"=TRUE ("Login")) -> ()  [unwired: 2 in, 2 out]
  n326 = while {
    tunnel: w99 -> [w800]
    tunnel: w98 -> [w799]
    tunnel: w94 -> [w797]
    tunnel: w90 -> [w795]
    shift-right: [w792] -> _
    shift-left: w95 -> [w798]
    shift-right: [w791] -> _
    shift-left: w91 -> [w796]
    shift-right: [w773] -> _
    shift-left: i8 0 -> [w794]
    tunnel: w85 -> [w780]
    shift-right: [w777] -> _
    shift-left: w86 -> [w784]
    shift-right: [w768] -> _
    shift-left: w81 -> [w771]
    tunnel: [w726] -> w38
    tunnel: [w725] -> w37
    tunnel: [w724] -> w36
    shift-right: [w714] -> _
    shift-left: w15 -> [w715]
    shift-right: [w696] -> _
    shift-left: w6 -> [w699]
    stop <- w724 stop-if-true
    # "Sensors reading"
    n327 = shared-variable ".\\setting Lib.lvlib\\ChannelSetting"() -> (w723:T7)  [unwired: 1 in, 1 out]
    n328 = property on="capture or not? 2" class="Bool (strict)"() -> ("Value"=w688:bool)  [unwired: 2 in, 2 out]
    n329 = flat-sequence {
      tunnel: w800 -> [w843]
      tunnel: w799 -> [w842]
      tunnel: [w841] -> w815
      tunnel: w798 -> [w841]
      tunnel: [w840] -> w814
      tunnel: w797 -> [w840]
      tunnel: [w839] -> w813
      tunnel: w796 -> [w839]
      tunnel: [w838] -> w812
      tunnel: w795 -> [w838]
      tunnel: [w837] -> w811
      tunnel: w794 -> [w837]
      tunnel: [w836] -> w785
      tunnel: w784 -> [w836]
      tunnel: [w835] -> w781
      tunnel: w780 -> [w835]
      tunnel: [w834] -> w772
      tunnel: w771 -> [w834]
      tunnel: [w827] -> w751
      tunnel: [w818] -> w738
      tunnel: [w826] -> w727
      tunnel: w723 -> [w825]
      tunnel: [w817] -> w722
      tunnel: [w819] -> w716
      tunnel: w715 -> [w819]
      tunnel: w699 -> [w816]
      tunnel: [w816] -> w697
      tunnel: w815 -> [w872]
      tunnel: w814 -> [w871]
      tunnel: w813 -> [w870]
      tunnel: w812 -> [w869]
      tunnel: [w868] -> w810
      tunnel: [w867] -> w809
      tunnel: [w847] -> w808
      tunnel: [w866] -> w807
      tunnel: w811 -> [w866]
      tunnel: [w865] -> w806
      tunnel: [w864] -> w786
      tunnel: w785 -> [w864]
      tunnel: [w863] -> w782
      tunnel: w781 -> [w863]
      tunnel: w772 -> [w862]
      tunnel: [w862] -> w769
      tunnel: [w861] -> w758
      tunnel: [w860] -> w757
      tunnel: [w859] -> w756
      tunnel: [w848] -> w755
      tunnel: [w858] -> w754
      tunnel: [w857] -> w753
      tunnel: [w856] -> w752
      tunnel: w751 -> [w849]
      tunnel: w738 -> [w854]
      tunnel: [w853] -> w737
      tunnel: [w852] -> w728
      tunnel: w727 -> [w852]
      tunnel: w722 -> [w851]
      tunnel: [w850] -> w717
      tunnel: w716 -> [w850]
      tunnel: [w847] -> w702
      tunnel: [w846] -> w698
      tunnel: w697 -> [w846]
      tunnel: w810 -> [w901]
      tunnel: w809 -> [w900]
      tunnel: w808 -> [w885]
      tunnel: w807 -> [w884]
      tunnel: w806 -> [w899]
      tunnel: [w901] -> w805
      tunnel: [w900] -> w804
      tunnel: [w885] -> w803
      tunnel: [w899] -> w802
      tunnel: [w882] -> w801
      tunnel: [w898] -> w787
      tunnel: w786 -> [w898]
      tunnel: [w897] -> w783
      tunnel: w782 -> [w897]
      tunnel: [w892] -> w779
      tunnel: [w878] -> w778
      tunnel: [w896] -> w770
      tunnel: w769 -> [w896]
      tunnel: w758 -> [w895]
      tunnel: w757 -> [w894]
      tunnel: w756 -> [w893]
      tunnel: w755 -> [w880]
      tunnel: w754 -> [w876]
      tunnel: w753 -> [w883]
      tunnel: w752 -> [w887]
      tunnel: [w873] -> w744
      tunnel: [w888] -> w743
      tunnel: [w875] -> w739
      tunnel: w737 -> [w891]
      tunnel: [w874] -> w736
      tunnel: [w890] -> w729
      tunnel: w728 -> [w890]
      tunnel: [w889] -> w718
      tunnel: w717 -> [w889]
      tunnel: w702 -> [w888]
      tunnel: w698 -> [w879]
      tunnel: [w881] -> w691
      tunnel: w688 -> [w873]
      tunnel: w805 -> [w921]
      tunnel: w804 -> [w920]
      tunnel: w803 -> [w914]
      tunnel: w802 -> [w913]
      tunnel: w801 -> [w911]
      tunnel: [w921] -> w790
      tunnel: [w920] -> w789
      tunnel: [w911] -> w788
      tunnel: w787 -> [w919]
      tunnel: w783 -> [w918]
      tunnel: w779 -> [w917]
      tunnel: w778 -> [w916]
      tunnel: [w915] -> w776
      tunnel: [w914] -> w775
      tunnel: [w913] -> w774
      tunnel: w770 -> [w912]
      tunnel: [w910] -> w767
      tunnel: [w910] -> w766
      tunnel: [w909] -> w745
      tunnel: w744 -> [w909]
      tunnel: w743 -> [w908]
      tunnel: [w907] -> w740
      tunnel: w739 -> [w907]
      tunnel: w736 -> [w906]
      tunnel: [w905] -> w735
      tunnel: [w904] -> w730
      tunnel: w729 -> [w904]
      tunnel: [w903] -> w719
      tunnel: w718 -> [w903]
      tunnel: [w902] -> w692
      tunnel: w691 -> [w902]
      tunnel: w790 -> [w939]
      tunnel: w789 -> [w938]
      tunnel: w788 -> [w929]
      tunnel: w776 -> [w937]
      tunnel: w775 -> [w936]
      tunnel: w774 -> [w932]
      tunnel: w767 -> [w935]
      tunnel: w766 -> [w933]
      tunnel: [w939] -> w765
      tunnel: [w938] -> w764
      tunnel: [w930] -> w763
      tunnel: [w937] -> w762
      tunnel: [w935] -> w761
      tunnel: [w933] -> w760
      tunnel: [w932] -> w759
      tunnel: w745 -> [w922]
      tunnel: [w928] -> w741
      tunnel: w740 -> [w928]
      tunnel: w735 -> [w927]
      tunnel: [w926] -> w734
      tunnel: [w925] -> w731
      tunnel: w730 -> [w925]
      tunnel: [w924] -> w720
      tunnel: w719 -> [w924]
      tunnel: [w923] -> w693
      tunnel: w692 -> [w923]
      tunnel: [w922] -> w690
      tunnel: w765 -> [w965]
      tunnel: w764 -> [w964]
      tunnel: w763 -> [w957]
      tunnel: w762 -> [w963]
      tunnel: w761 -> [w962]
      tunnel: w760 -> [w961]
      tunnel: w759 -> [w958]
      tunnel: [w965] -> w750
      tunnel: [w964] -> w749
      tunnel: [w957] -> w748
      tunnel: [w963] -> w747
      tunnel: [w962] -> w746
      tunnel: [w951] -> w742
      tunnel: w741 -> [w951]
      tunnel: w734 -> [w950]
      tunnel: [w944] -> w733
      tunnel: [w949] -> w732
      tunnel: w731 -> [w949]
      tunnel: [w945] -> w721
      tunnel: w720 -> [w945]
      tunnel: [w942] -> w694
      tunnel: w693 -> [w942]
      tunnel: w690 -> [w940]
      tunnel: [w940] -> w689
      tunnel: w732 -> [w980]
      tunnel: w733 -> [w974]
      tunnel: w742 -> [w977]
      tunnel: w750 -> [w985]
      tunnel: w749 -> [w984]
      tunnel: w748 -> [w983]
      tunnel: w747 -> [w982]
      tunnel: w746 -> [w981]
      tunnel: w721 -> [w979]
      tunnel: [w985] -> w713
      tunnel: [w984] -> w712
      tunnel: [w983] -> w711
      tunnel: [w982] -> w710
      tunnel: [w981] -> w709
      tunnel: [w973] -> w708
      tunnel: [w980] -> w707
      tunnel: [w978] -> w706
      tunnel: [w975] -> w705
      tunnel: [w975] -> w704
      tunnel: [w976] -> w701
      tunnel: [w975] -> w700
      tunnel: [w972] -> w695
      tunnel: w694 -> [w972]
      tunnel: w689 -> [w967]
      tunnel: [w996] -> w714
      tunnel: [w997] -> w726
      tunnel: [w987] -> w725
      tunnel: [w998] -> w768
      tunnel: [w999] -> w777
      tunnel: [w1000] -> w773
      tunnel: [w1001] -> w791
      tunnel: [w1002] -> w792
      tunnel: w713 -> [w1002]
      tunnel: w712 -> [w1001]
      tunnel: w711 -> [w1000]
      tunnel: w710 -> [w999]
      tunnel: w709 -> [w998]
      tunnel: w708 -> [w988]
      tunnel: w707 -> [w997]
      tunnel: w706 -> [w996]
      tunnel: w705 -> [w995]
      tunnel: w704 -> [w994]
      tunnel: [w993] -> w703
      tunnel: w701 -> [w989]
      tunnel: w700 -> [_]
      tunnel: [w986] -> w696
      tunnel: w695 -> [w986]
      frame #0 {
        # "sensor data read"
        n330 = Unbundle By Name(w825) -> ("ch sensor1"=w824:dbl, "ch sensor2"=w823:dbl, "chs ensor3"=w822:dbl, "ch sw sensor1"=w821:dbl, "ch sw sensor2"=w820:dbl)
        n331 = call "adamread.vi"("TCP Connection Refnum in"=w843, "error in (no error)"=w842) -> ("TCP Connection Refnum (dup)"=w826:refnum<k5>, "Slave Input Registers 2"=w833:dbl[], "error out 2"=w818:errorcluster)  [unwired: 11 in]
        n332 = case shown="Error .." w818 {
          tunnel: [FALSE ("error?") TRUE ("error?")] -> w817
          frame No Error {
          }
          frame Error {
          }
        }
        n333 = Index Array(array=w833, index #1=w824, index #2=w823, index #3=w822, index #4=w821, index #5=w820) -> (element #1=w832:dbl, element #2=w831:dbl, element #3=w830:dbl, element #4=w829:dbl, element #5=w828:dbl)
        n334 = Build Array(w832, w831, w830, w829, w828) -> (w827:dbl[])
      }
      frame #1 {
        # "Averaging of sesor pallet"
        n335 = shared-variable ".\\setting Lib.lvlib\\CurvSetting"(error in=w854) -> (w855:T8, error out=w853:errorcluster)
        n336 = shared-variable ".\\setting Lib.lvlib\\RisingSensorThr"() -> (w856:dbl[])  [unwired: 1 in, 1 out]
        n337 = call "Waveform Averaging.vi"("2D curv array in"=w872, "array sensor in"=w849, "avg wind1"=w871, "2D Sw Array In"=w870, "avg Win2"=w869) -> ("2D curv Array out"=w868:dbl[][], "2D Sw Array Out"=w867:dbl[][], "Curv Average Array Out"=w847:dbl[], "SW Average Array Out"=w865:dbl[])  [unwired: 11 in]
        n338 = property on="machine pallet speed" class="DigNum (strict)"() -> ("Value"=w848:dbl)  [unwired: 2 in, 2 out]
        n339 = Unbundle By Name(w855) -> ("low level read thr 1"=w861:dbl, "low level read thr 2"=w860:dbl, "low level read thr 3"=w859:dbl, "falling level thr"=w858:dbl, "counting role 2"=w857:T9)  [unwired: 1 out]
        "Sen.ER" <- w851
      }
      frame #2 {
        # "count coloumns and pallet"
        n340 = Build Array(w895, w894, w893) -> (w892:dbl[])
        n341 = property on="capture or not?" class="Bool (strict)"(error in=w891) -> (error out=w877:errorcluster, "Value"=w886:bool)  [unwired: 1 in, 1 out]
        n342 = call "sensor count.vi"("sensor thr array"=w887, "pallet speed"=w880, "speed array in"=w879, "capture y or no ?"=w886, "sensor data"=w885, "counter input"=w884, "counting role"=w883, "error in"=w877, "falling level thr"=w876) -> ("column count"=w878:bool, "speed array out"=w881:dbl[], "counter out"=w882:i8, "pallet detect"=w875:bool, "error out"=w874:errorcluster)  [unwired: 2 out]
        "Col. Count" <- w878
      }
      frame #3 {
        # "Curv Measuement"
        n343 = call "curvness detection.vi"("2D curv array in"=w919, "array sensor in"=w908, "avg wind1"=w918, "min level thr"=w917, "coloumn count"=w916, "curv Array"=w912, "col count"=w911, "error in (no error)"=w906) -> ("2D curv array Out"=w915:dbl[][], "curv Array out"=w910:dbl[], "error out"=w905:errorcluster)  [unwired: 8 in, 1 out]
      }
      frame #4 {
        # "Trends Show"
        n344 = property on="Sen Plt\nNUM" class="DigNum (strict)"(error in=w927) -> (error out=w926:errorcluster, "Value"=w934:i16)  [unwired: 1 in, 1 out]
        n345 = Select(t=i8 0, s=w922, f=w929) -> (s? t:f=w930:i8)
        "Col\n NUM" <- w930
        n346 = call "waveform show.vi"("curv array in"=w936, "SW array in"=w932, "Col Count 2"=w929, "coloumn curvness array"=w933, "Sensor Pallet NUM 2"=w934) -> ()  [unwired: 15 in]
      }
      frame #5 {
        # "SideWall and Curvensee situation set \nSideWall and Curvness situation set"
        n347 = shared-variable ".\\setting Lib.lvlib\\SW&CurvSetting"(error in=w950) -> (w955:T10, error out=w941:errorcluster)
        n348 = Index Array(array=w961, index=5) -> (element=w959:dbl)
        "CURV (mm)" <- w959
        n349 = property on="GB sit 2" class="DigNum (strict)"() -> ("Value"=w948:i8)  [unwired: 2 in, 2 out]
        n350 = call "sW&col situation.vi"("Overal CURV(mm)"=w959, "SW array in"=w958, "curv and Sw setting"=w955, "col count"=w957, "capture"=w940, "error in (no error)"=w941) -> ("curv sit"=w954:bool, "right SideWall"=w953:bool, "Left SideWall"=w952:bool, "error out"=w944:errorcluster)  [unwired: 9 in, 1 out]
        "curv sit" <- w954
        "SWL 2" <- w952
        "SWR 2" <- w953
        n351 = Equal?(x=w948, y=i8 2) -> (x = y?=w946:bool)
        n352 = Bundle("curv sit"=w954, "right SideWall"=w953, "Left SideWall"=w952) -> (→"SW&col sit":T11)  [unwired: 1 in]
        n353 = Compound Arithmetic op=OR(w954, w953, w952, w946) -> (w943:bool)
        n354 = case shown="True" w943 {
          tunnel: w943 -> [_ _]
          frame False {
          }
          frame True {
            w966 = TRUE
            n355 = property on="Alarm" class="Bool (strict)"("Blinking"=w966) -> ()  [unwired: 2 in, 2 out]
            n356 = property on="Alarm" class="Bool (strict)"("Value"=w966) -> ()  [unwired: 2 in, 2 out]
          }
        }
        "curv Array out" <- w961
      }
      frame #6 {
        n357 = property on="capture or not?" class="Bool (strict)"() -> ("Value"=w971:bool)  [unwired: 2 in, 2 out]
        n358 = property on="machine pallet speed" class="DigNum (strict)"() -> ("Value"=w970:dbl)  [unwired: 2 in, 2 out]
        n359 = call "speed&col syncroun 2.vi"("speed array in"=w979, "speed"=w970, "width"=1.6, "start"=w971, "instant capture"=w967, "acceptable width"=1.2, "plt count"=w977, "error in (no error)"=w974) -> ("total movement"=w976:dbl, "speed array out"=w978:dbl[], "plt count accept"=w975:bool, "error out"=w973:errorcluster)  [unwired: 6 in, 2 out]
        "Plt Count" <- w977
      }
      frame #7 {
        n360 = call "Elapsed Time"("Reset"=w995, "error in (no error)"=w988) -> ("Elapsed Time (s)"=w992:dbl, "error out"=w987:errorcluster)  [unwired: 10 in, 6 out]
        n361 = Greater Or Equal?(x=w992, y=1.0) -> (x >= y?=w990:bool)
        n362 = case shown="False" w994 {
          tunnel: [w1003 TRUE] -> w993
          tunnel: w990 -> [w1004 _]
          frame False {
            n363 = case shown="True" w1004 {
              tunnel: [w1005 FALSE ("Value")] -> w1003
              frame False {
                n364 = property on="pallet count accept" class="Bool (strict)"() -> ("Value"=w1005:bool)  [unwired: 2 in, 2 out]
              }
              frame True {
              }
            }
          }
          frame True {
          }
        }
        "pallet Movement (m)" <- w989
      }
    }
    n365 = Wait (ms)(milliseconds to wait=u32 10) -> ()  [unwired: 1 out]
    n366 = shared-variable ".\\setting Lib.lvlib\\StopOk"() -> (w724:bool)  [unwired: 1 in, 1 out]
    "pallet count accept" <- w703
    "Plt Count 2" <- w703
    "error out 6" <- w725
  }
  "sensor loop stop" <- w36
  n367 = while {
    shift-right: [w1024] -> _
    shift-left: 0 -> [w1025]
    shift-right: [w1023] -> _
    shift-left: w102 -> [w1027]
    shift-right: [w1016] -> _
    shift-left: 0 -> [w1021]
    tunnel: w77 -> [w1019]
    tunnel: w73 -> [w1018]
    tunnel: w72 -> [w1017]
    tunnel: [w1015] -> w71
    tunnel: w67 -> [w1014]
    shift-right: [w1010] -> _
    shift-left: w63 -> [w1013]
    tunnel: w75 -> [w1020]
    tunnel: [w1009] -> w58
    tunnel: w101 -> [w1026]
    tunnel: [w1022] -> w21
    tunnel: [w1008] -> w34
    stop <- w1008 stop-if-true
    # "Main Loop"
    n368 = event shown="[0] Timeout" {
      selector: _ -> [_ _]
      dyn-events: _ -> [_ _]
      timeout: 0 -> [_ _]
      tunnel: w1027 -> [w1059 w1536]
      tunnel: w1026 -> [w1058 w1535]
      tunnel: w1025 -> [w1057 w1531]
      tunnel: [w1056 w1531] -> w1024
      tunnel: [w1055 w1534] -> w1023
      tunnel: [w1054 w1533] -> w1022
      tunnel: w1021 -> [w1052 w1532]
      tunnel: w1020 -> [w1051 w1524]
      tunnel: w1019 -> [w1050 w1530]
      tunnel: w1018 -> [w1049 _]
      tunnel: w1017 -> [w1048 _]
      tunnel: [w1047 w1532] -> w1016
      tunnel: [w1046 w1530] -> w1015
      tunnel: w1014 -> [w1045 _]
      tunnel: w1013 -> [w1044 w1529]
      tunnel: [w1043 w1528] -> w1010
      tunnel: [w1035 w1523] -> w1009
      event Timeout {
        w1029 = u16 1 items=["Falling Edge", "Rising Edge"] ("trigger slope")
        n369 = event-data() -> ()  [unwired: 1 in, 3 out]
        n370 = shared-variable ".\\setting Lib.lvlib\\General Setting"() -> (w1038:T6)  [unwired: 1 in, 1 out]
        n371 = Get Date/Time In Seconds() -> (seconds since 1Jan1904=w1042:timestamp)
        n372 = property on="pallet count accept" class="Bool (strict)"() -> ("Value"=w1031:bool)  [unwired: 2 in, 2 out]
        n373 = Boolean To (0,1)(Boolean=w1031) -> (0, 1=w1032:i16)
        n374 = property on="capture or not? 2" class="Bool (strict)"() -> ("Value"=w1028:bool)  [unwired: 2 in, 2 out]
        n375 = Get Date/Time String(seconds (now)=w1042, want seconds? (F)=TRUE) -> (date string=→"time&date 2":string, time string=→"time&date":string)  [unwired: 1 in]
        n376 = Build Array(w1032) -> (w1033:i16[])
        n377 = call-poly <vilib>:"Basic Level Trigger Detection.vi"("signal in"=w1033, "level"=0.5, "trigger slope"=w1029) -> ("trigger detected?"=w1030:bool)  [unwired: 10 in, 2 out]
        n378 = Unbundle By Name(w1038) -> ("madule path"=w1037:path, "Img Path"=w1036:path)
        n379 = Or(x=w1030, y=w1028) -> (x .or. y?=w1053:bool)
        n380 = case shown="True" w1053 {
          tunnel: w1059 -> [w1065 w1204]
          tunnel: w1058 -> [w1064 w1203]
          tunnel: [w1065 w1202] -> w1055
          tunnel: [w1064 w1201] -> w1054
          tunnel: w1057 -> [w1066 w1200]
          tunnel: [w1066 w1199] -> w1056
          tunnel: w1052 -> [w1063 w1198]
          tunnel: w1051 -> [w1060 w1195]
          tunnel: w1050 -> [w1062 w1186]
          tunnel: w1049 -> [_ w1183]
          tunnel: w1048 -> [_ w1181]
          tunnel: [w1063 w1175] -> w1047
          tunnel: [w1062 w1172] -> w1046
          tunnel: w1045 -> [_ w1171]
          tunnel: w1044 -> [w1061 w1167]
          tunnel: [w1061 w1122] -> w1043
          tunnel: w1037 -> [_ w1097]
          tunnel: w1036 -> [_ w1095]
          tunnel: [w1060 w1076] -> w1035
          frame False {
          }
          frame True {
            n381 = flat-sequence {
              tunnel: w1200 -> [w1220]
              tunnel: w1203 -> [w1221]
              tunnel: w1204 -> [w1222]
              tunnel: [w1222] -> w1210
              tunnel: [w1221] -> w1209
              tunnel: [w1220] -> w1208
              tunnel: w1198 -> [w1219]
              tunnel: [w1218] -> w1197
              tunnel: w1195 -> [w1217]
              tunnel: [w1217] -> w1193
              tunnel: [w1216] -> w1187
              tunnel: w1186 -> [w1216]
              tunnel: [w1215] -> w1184
              tunnel: w1183 -> [w1215]
              tunnel: [w1214] -> w1182
              tunnel: w1181 -> [w1214]
              tunnel: w1171 -> [w1213]
              tunnel: [w1213] -> w1168
              tunnel: [w1212] -> w1098
              tunnel: w1097 -> [w1212]
              tunnel: [w1211] -> w1096
              tunnel: w1095 -> [w1211]
              tunnel: [w1240] -> w1207
              tunnel: [w1237] -> w1206
              tunnel: [w1236] -> w1205
              tunnel: w1210 -> [w1248]
              tunnel: w1209 -> [w1254]
              tunnel: w1208 -> [w1241]
              tunnel: w1197 -> [w1232]
              tunnel: [w1231] -> w1196
              tunnel: [w1230] -> w1194
              tunnel: w1193 -> [w1230]
              tunnel: [w1229] -> w1188
              tunnel: w1187 -> [w1229]
              tunnel: w1184 -> [w1228]
              tunnel: w1182 -> [w1227]
              tunnel: [w1228] -> w1179
              tunnel: [w1227] -> w1177
              tunnel: [w1226] -> w1173
              tunnel: [w1225] -> w1169
              tunnel: w1168 -> [w1225]
              tunnel: [w1224] -> w1100
              tunnel: w1098 -> [w1224]
              tunnel: w1096 -> [w1223]
              tunnel: [w1223] -> w1093
              tunnel: w1207 -> [w1300]
              tunnel: w1206 -> [w1299]
              tunnel: w1205 -> [w1298]
              tunnel: w1196 -> [_]
              tunnel: w1194 -> [w1291]
              tunnel: [w1300] -> w1192
              tunnel: [w1299] -> w1191
              tunnel: [w1298] -> w1190
              tunnel: [w1297] -> w1189
              tunnel: w1188 -> [w1297]
              tunnel: [w1287] -> w1185
              tunnel: [w1296] -> w1180
              tunnel: w1179 -> [w1296]
              tunnel: [w1295] -> w1178
              tunnel: w1177 -> [w1295]
              tunnel: [w1292] -> w1176
              tunnel: [w1294] -> w1174
              tunnel: w1173 -> [w1294]
              tunnel: [w1293] -> w1170
              tunnel: w1169 -> [w1293]
              tunnel: [w1290] -> w1101
              tunnel: w1100 -> [w1289]
              tunnel: [w1289] -> w1099
              tunnel: [w1288] -> w1094
              tunnel: w1093 -> [w1288]
              tunnel: [w1324] -> w1166
              tunnel: [w1323] -> w1165
              tunnel: [w1322] -> w1164
              tunnel: [w1321] -> w1163
              tunnel: [w1320] -> w1162
              tunnel: [w1319] -> w1161
              tunnel: [w1318] -> w1160
              tunnel: [w1305] -> w1159
              tunnel: w1170 -> [_]
              tunnel: w1174 -> [w1321]
              tunnel: w1176 -> [w1313]
              tunnel: w1178 -> [w1314]
              tunnel: w1180 -> [w1315]
              tunnel: w1185 -> [w1316]
              tunnel: w1189 -> [w1317]
              tunnel: w1190 -> [w1322]
              tunnel: w1191 -> [w1323]
              tunnel: w1192 -> [w1324]
              tunnel: [w1312] -> w1148
              tunnel: w1101 -> [w1311]
              tunnel: w1099 -> [w1309]
              tunnel: w1094 -> [w1308]
              tunnel: [w1308] -> w1091
              tunnel: [w1307] -> w1087
              tunnel: w1166 -> [w1346]
              tunnel: w1165 -> [w1345]
              tunnel: w1164 -> [w1344]
              tunnel: w1163 -> [w1343]
              tunnel: w1162 -> [w1342]
              tunnel: w1161 -> [w1340]
              tunnel: [w1346] -> w1158
              tunnel: [w1345] -> w1157
              tunnel: [w1344] -> w1156
              tunnel: [w1343] -> w1155
              tunnel: [w1342] -> w1154
              tunnel: [w1338] -> w1153
              tunnel: [w1337] -> w1152
              tunnel: w1160 -> [w1337]
              tunnel: [w1336] -> w1151
              tunnel: w1159 -> [w1336]
              tunnel: [w1335] -> w1150
              tunnel: [w1334] -> w1149
              tunnel: w1148 -> [w1334]
              tunnel: [w1333] -> w1147
              tunnel: [w1327] -> w1114
              tunnel: [w1326] -> w1092
              tunnel: w1091 -> [w1326]
              tunnel: [w1325] -> w1088
              tunnel: w1087 -> [w1325]
              tunnel: w1158 -> [w1375]
              tunnel: [w1375] -> w1146
              tunnel: w1157 -> [w1374]
              tunnel: [w1374] -> w1144
              tunnel: w1156 -> [w1373]
              tunnel: [w1373] -> w1142
              tunnel: w1155 -> [w1372]
              tunnel: [w1372] -> w1140
              tunnel: w1154 -> [w1371]
              tunnel: [w1371] -> w1138
              tunnel: w1153 -> [w1370]
              tunnel: [w1370] -> w1136
              tunnel: [w1355] -> w1134
              tunnel: w1152 -> [w1369]
              tunnel: [w1369] -> w1132
              tunnel: w1151 -> [w1368]
              tunnel: [w1368] -> w1130
              tunnel: w1150 -> [w1347]
              tunnel: w1149 -> [w1363]
              tunnel: w1147 -> [w1362]
              tunnel: [w1361] -> w1124
              tunnel: w1114 -> [w1359]
              tunnel: [w1351] -> w1103
              tunnel: [w1350] -> w1102
              tunnel: w1092 -> [w1349]
              tunnel: [w1348] -> w1089
              tunnel: w1088 -> [w1348]
              tunnel: w1146 -> [w1397]
              tunnel: [w1397] -> w1145
              tunnel: w1144 -> [w1396]
              tunnel: [w1396] -> w1143
              tunnel: w1142 -> [w1395]
              tunnel: [w1395] -> w1141
              tunnel: w1140 -> [w1394]
              tunnel: [w1394] -> w1139
              tunnel: w1138 -> [w1393]
              tunnel: [w1393] -> w1137
              tunnel: w1136 -> [w1392]
              tunnel: [w1392] -> w1135
              tunnel: w1134 -> [w1391]
              tunnel: [w1391] -> w1133
              tunnel: w1132 -> [w1390]
              tunnel: [w1390] -> w1131
              tunnel: w1130 -> [w1389]
              tunnel: [w1389] -> w1129
              tunnel: [w1388] -> w1128
              tunnel: [w1383] -> w1127
              tunnel: [w1382] -> w1126
              tunnel: [w1381] -> w1125
              tunnel: w1124 -> [w1380]
              tunnel: [w1379] -> w1123
              tunnel: w1103 -> [w1378]
              tunnel: w1102 -> [w1377]
              tunnel: [w1376] -> w1090
              tunnel: w1089 -> [w1376]
              tunnel: w1145 -> [w1449]
              tunnel: w1143 -> [w1448]
              tunnel: w1141 -> [w1447]
              tunnel: w1139 -> [w1446]
              tunnel: w1137 -> [w1445]
              tunnel: w1135 -> [w1404]
              tunnel: w1167 -> [w1444]
              tunnel: w1133 -> [w1407]
              tunnel: w1131 -> [w1430]
              tunnel: w1129 -> [w1429]
              tunnel: w1128 -> [w1428]
              tunnel: w1127 -> [w1414]
              tunnel: w1126 -> [w1413]
              tunnel: w1125 -> [w1412]
              tunnel: w1123 -> [w1411]
              tunnel: [w1449] -> w1121
              tunnel: [w1448] -> w1120
              tunnel: [w1447] -> w1119
              tunnel: [w1446] -> w1118
              tunnel: [w1445] -> w1117
              tunnel: [w1410] -> w1116
              tunnel: [w1409] -> w1115
              tunnel: [w1404] -> w1113
              tunnel: [w1407] -> w1112
              tunnel: w1090 -> [w1399]
              tunnel: w1121 -> [w1480]
              tunnel: w1120 -> [w1484]
              tunnel: w1119 -> [w1483]
              tunnel: w1118 -> [w1482]
              tunnel: w1117 -> [w1481]
              tunnel: w1116 -> [w1476]
              tunnel: w1115 -> [w1455]
              tunnel: w1113 -> [w1451]
              tunnel: w1112 -> [w1450]
              tunnel: [w1480] -> w1111
              tunnel: [w1484] -> w1110
              tunnel: [w1483] -> w1109
              tunnel: [w1482] -> w1108
              tunnel: [w1481] -> w1107
              tunnel: [w1454] -> w1106
              tunnel: [w1462] -> w1105
              tunnel: [w1461] -> w1104
              tunnel: [w1451] -> w1079
              tunnel: [w1450] -> w1078
              tunnel: w1111 -> [w1501]
              tunnel: w1110 -> [w1500]
              tunnel: w1109 -> [w1499]
              tunnel: w1108 -> [w1498]
              tunnel: w1107 -> [w1497]
              tunnel: w1106 -> [w1496]
              tunnel: w1105 -> [w1489]
              tunnel: w1104 -> [w1495]
              tunnel: [w1501] -> w1086
              tunnel: [w1500] -> w1085
              tunnel: [w1499] -> w1084
              tunnel: [w1498] -> w1083
              tunnel: [w1497] -> w1082
              tunnel: [w1496] -> w1081
              tunnel: [w1488] -> w1080
              tunnel: w1079 -> [w1488]
              tunnel: w1078 -> [w1487]
              tunnel: [w1487] -> w1077
              tunnel: [w1486] -> w1075
              tunnel: [w1485] -> w1074
              tunnel: w1086 -> [w1513]
              tunnel: w1085 -> [w1512]
              tunnel: w1084 -> [w1511]
              tunnel: w1083 -> [w1510]
              tunnel: w1082 -> [w1509]
              tunnel: w1081 -> [w1508]
              tunnel: w1080 -> [w1507]
              tunnel: w1077 -> [w1506]
              tunnel: w1075 -> [w1504]
              tunnel: w1074 -> [w1502]
              tunnel: [w1513] -> w1073
              tunnel: [w1512] -> w1072
              tunnel: [w1511] -> w1071
              tunnel: [w1510] -> w1070
              tunnel: [w1509] -> w1069
              tunnel: [w1508] -> w1068
              tunnel: [w1505] -> w1067
              tunnel: [w1515] -> w1076
              tunnel: [w1516] -> w1122
              tunnel: [w1517] -> w1172
              tunnel: [w1518] -> w1175
              tunnel: [w1519] -> w1199
              tunnel: [w1520] -> w1201
              tunnel: [w1521] -> w1202
              tunnel: w1073 -> [w1521]
              tunnel: w1072 -> [w1520]
              tunnel: w1071 -> [w1519]
              tunnel: w1070 -> [w1518]
              tunnel: w1069 -> [w1517]
              tunnel: w1068 -> [w1516]
              tunnel: w1067 -> [w1515]
              frame #0 {
                n382 = Increment(x=w1219) -> (x+1=w1218:i32)
              }
              frame #1 {
                # "rotate label"
                n383 = for {
                  tunnel: w1248 -> [w1286] mode=indexing
                  tunnel: w1254 -> [w1285] mode=indexing
                  tunnel: [w1281] -> w1251 mode=indexing
                  tunnel: [w1280] -> w1249 mode=indexing
                  tunnel: [w1279] -> w1247 mode=indexing
                  tunnel: [w1278] -> w1246 mode=indexing
                  tunnel: [w1277] -> w1238 mode=indexing
                  n384 = property class="Bool"(reference=w1286, error in=w1285) -> (reference out=w1284:refnum<vi>, error out=w1283:errorcluster, "BoolText.Text"=w1278:string)
                  n385 = property class="Bool"(reference=w1284, error in=w1283) -> (reference out=w1279:refnum<vi>, error out=w1277:errorcluster, "Colors [4]"=w1280:cluster{u32, u32}[])
                  n386 = Index Array(array=w1280, index=0) -> (element=w1281:cluster{u32, u32})
                }
                n387 = Greater?(x=w1232, y=232) -> (0:w1235:bool)
                n388 = Select(t=1, s=w1235, f=w1232) -> (s? t:f=w1226:i32)
                n389 = Number To Decimal String(number=w1226) -> (decimal integer string=w1231:string)  [unwired: 1 in]
                n390 = Rotate 1D Array(1:w1246, 2:1 ("n")) -> (0:w1245:string[])
                n391 = Rotate 1D Array(1:w1251, 2:1 ("n")) -> (0:w1250:cluster{u32, u32}[])
                n392 = for {
                  tunnel: w1250 -> [w1276] mode=indexing
                  tunnel: w1249 -> [w1274] mode=indexing
                  tunnel: w1247 -> [w1273] mode=indexing
                  tunnel: w1245 -> [w1271] mode=indexing
                  tunnel: [w1269] -> w1242 mode=indexing
                  tunnel: [w1268] -> w1239 mode=indexing
                  tunnel: w1238 -> [w1267] mode=indexing
                  n393 = property class="Bool"(reference=w1273, error in=w1267, "BoolText.Text"=w1271) -> (reference out=w1272:refnum<vi>, error out=w1266:errorcluster)
                  n394 = Replace Array Subset(array=w1274, new element=w1276, index=0) -> (w1270:cluster{u32, u32}[])
                  n395 = property class="Bool"(reference=w1272, error in=w1266, "Colors [4]"=w1270) -> (reference out=w1269:refnum<vi>, error out=w1268:errorcluster)
                }
                n396 = Greater?(x=w1241, y=231) -> (0:w1243:bool)
                n397 = case shown="False" w1243 {
                  tunnel: w1242 -> [w1262 w1265]
                  tunnel: w1241 -> [w1258 w1263]
                  tunnel: [w1257 w1265] -> w1240
                  tunnel: w1239 -> [w1256 w1264]
                  tunnel: [w1256 w1264] -> w1237
                  tunnel: [w1255 w1263] -> w1236
                  frame False {
                    n398 = Increment(x=w1258) -> (x+1=w1255:i32)
                    n399 = Index Array(array=w1262, index=w1258) -> (element=w1261:refnum<vi>)
                    n400 = property class="Bool"(reference=w1261, "DisabledEnum"=T4."Enabled" ("Disabled")) -> (reference out=w1259:refnum<vi>)  [unwired: 1 in, 1 out]
                    n401 = Replace Array Subset(array=w1262, new element=w1259, index=w1258) -> (w1257:refnum<vi>[])
                  }
                  frame True {
                  }
                }
              }
              frame #2 {
                n402 = shared-variable ".\\setting Lib.lvlib\\GratbarSetting"() -> (w1292:T12)  [unwired: 1 in, 1 out]
                n403 = property on="snap img" class="IMAQImage (strict)"(error in=w1291) -> (error out=w1290:errorcluster, "Value"=w1287:T1)  [unwired: 1 in, 1 out]
              }
              frame #3 {
                # "gratebar defect detection"
                n404 = call "pyton dpallet car test.vi"("session in"=w1317, "module path 2"=w1309, "function name"="find_defects", "Image Src"=w1316, "img crop"=w1315, "img out"=w1314, "image setting cluster in"=w1313, "error in (no error)"=w1311) -> ("frm false"=w1307:bool, "Image Display"=w1312:T1, "session out"=w1320:refnum<k35>, "error out"=w1319:errorcluster, "Defect Ratio"=w1318:dbl, "defect type"=w1305:dbl)  [unwired: 5 in, 1 out]
                "Pallet Defects View" <- w1312
                "GB defects%" <- w1318
                "Frm False" <- w1307
                n405 = Greater?(x=w1305, y=1.0) -> (0:w1306:bool)
                n406 = Select(t="hole", s=w1306, f="gap" ("DEF TYPE")) -> (s? t:f=→"DEF TYPE":string)
              }
              frame #4 {
                w1331 = 232 ("y")
                # "palet and curv number creation"
                n407 = control-ref of="232"() -> (w1341:refnum<vi>)
                n408 = property class="Bool"(reference=w1341, error in=w1340) -> (error out=w1333:errorcluster, "BoolText.Text"=w1335:string)  [unwired: 1 out]
                "PLT NUM :" <- w1335
                n409 = Decimal String To Number(string=w1335) -> (number=w1332:i32)  [unwired: 2 in, 1 out]
                n410 = Add(x=w1332, y=45) -> (x+y=w1328:i32)
                n411 = Decrement(x=w1332) -> (x-1=w1338:i32)
                n412 = Greater?(x=w1328, y=w1331) -> (0:w1330:bool)
                n413 = Subtract(x=w1328, y=w1331) -> (x-y=w1329:i32)
                n414 = Select(t=w1329, s=w1330, f=w1328) -> (s? t:f=w1327:i32)
                "Sen Plt\nNUM" <- w1327
              }
              frame #5 {
                # "IMG SAVE"
                n415 = shared-variable ".\\setting Lib.lvlib\\PalletGratbarThrArray"() -> (w1354:u16[])  [unwired: 1 in, 1 out]
                n416 = Subtract(x=w1359, y=2) -> (x-y=w1356:i32)
                n417 = Concatenate Strings("pallet_p(" ("string"), w1347, ").bmp" ("string")) -> (w1365:string)
                n418 = Less Than 0?(x=w1356) -> (x < 0?=w1358:bool)
                n419 = Build Path(base path=w1349, name or relative path=w1365) -> (appended path=w1364:path)
                n420 = Select(t=u16 231, s=w1358, f=w1356) -> (s? t:f=w1355:i32)
                n421 = call-poly "IMAQ Write File 2"("error in (no error)"=w1362, "File Path"=w1364, "Image"=w1363) -> ("error out"=w1361:errorcluster)  [unwired: 7 in, 1 out]
                n422 = Index Array(array=w1354, index #1=0 ("index"), index #2=1 ("index")) -> (element #1=w1351:u16, element #2=w1350:u16)
              }
              frame #6 {
                # "GRATE BAR SITUATION"
                n423 = property on="SW&col sit" class="Clust (strict)"(error in=w1380) -> (error out=w1379:errorcluster, "Value"=w1387:T2)  [unwired: 1 in, 1 out]
                n424 = Unbundle By Name(w1387) -> ("curv sit"=w1386:bool, "Right Sidewall"=w1385:bool, "Left SideWall"=w1384:bool)
                n425 = call "GB Situation.vi"("GB defects"=w1390, "def type"=w1389, "thr1"=w1378, "thr2"=w1377) -> ("GB sit"=w1388:i8)  [unwired: 11 in]
                "GB sit 2" <- w1388
                n426 = Boolean To (0,1)(Boolean=w1386) -> (0, 1=w1383:i16)
                n427 = Boolean To (0,1)(Boolean=w1385) -> (0, 1=w1382:i16)
                n428 = Boolean To (0,1)(Boolean=w1384) -> (0, 1=w1381:i16)
              }
              frame #7 {
                # "SAVE TO INFO ARRAY"
                n429 = Boolean To (0,1)(Boolean=w1399) -> (0, 1=w1398:i16)
                n430 = property on="curv Array out" class="Arr (strict)"(error in=w1411) -> (error out=w1410:errorcluster, "Value"=w1423:dbl[])  [unwired: 1 in, 1 out]
                n431 = property on="Sync" class="Bool (strict)"() -> ("Value"=w1402:bool)  [unwired: 2 in, 2 out]
                n432 = Boolean To (0,1)(Boolean=w1402) -> (0, 1=w1401:i16)
                n433 = Index Array(array=w1423, index #1=0 ("index"), index #2=1 ("index"), index #3=2 ("index"), index #4=3 ("index"), index #5=4 ("index"), index #6=5 ("index")) -> (element #1=w1415:dbl, element #2=w1416:dbl, element #3=w1417:dbl, element #4=w1418:dbl, element #5=w1419:dbl, element #6=w1420:dbl)
                n434 = Increment(x=w1404) -> (x+1=w1405:i32)
                n435 = Replace Array Subset(array=w1444, new element #1=w1430, index (row) #1=w1404, index (col) #1=0 ("disabled index (col)"), new element #2=w1429, index (row) #2=w1404, index (col) #2=1 ("disabled index (col)"), new element #3=w1428, index (row) #3=w1404, index (col) #3=2 ("disabled index (col)"), new element #4=w1420, index (row) #4=w1407, index (col) #4=3 ("disabled index (col)"), new element #5=w1414, index (row) #5=w1407, index (col) #5=4 ("disabled index (col)"), new element #6=w1413, index (row) #6=w1407, index (col) #6=5 ("disabled index (col)"), new element #7=w1412, index (row) #7=w1407, index (col) #7=6 ("disabled index (col)"), new element #8=0.0 ("new element/subarray"), index (row) #8=w1407, index (col) #8=7 ("disabled index (col)"), new element #9=w1415, index (row) #9=w1407, index (col) #9=8 ("disabled index (col)"), new element #10=w1416, index (row) #10=w1407, index (col) #10=9 ("disabled index (col)"), new element #11=w1417, index (row) #11=w1407, index (col) #11=10 ("disabled index (col)"), new element #12=w1418, index (row) #12=w1407, index (col) #12=11 ("disabled index (col)"), new element #13=w1419, index (row) #13=w1407, index (col) #13=12 ("disabled index (col)"), new element #14=w1405, index (row) #14=w1404, index (col) #14=13 ("disabled index (col)"), new element #15=w1401, index (row) #15=w1404, index (col) #15=14 ("disabled index (col)"), new element #16=w1398, index (row) #16=w1404, index (col) #16=15 ("disabled index (col)")) -> (w1409:dbl[][])
              }
              frame #8 {
                # "PALLET LABELING"
                n436 = Index Array(array=w1480, index #1=0 ("index"), index #2=188 ("index")) -> (element #1=w1477:refnum<vi>, element #2=w1470:refnum<vi>)
                n437 = call "pallet labeling 2.vi"("Array"=w1455, "plt num"=w1451, "curv num"=w1450) -> ("pallet situation"=w1452:i16, "camera pallet color"=w1473:cluster{u32, u32}, "sensor pallet color"=w1466:cluster{u32, u32}, "gb color"=w1460:cluster{u32, u32})  [unwired: 12 in, 1 out]
                n438 = property class="Bool"(reference=w1477, error in=w1476) -> (reference out=w1472:refnum<vi>, error out=w1456:errorcluster, "Colors [4]"=w1475:cluster{u32, u32}[])
                n439 = Cluster To Array(cluster=w1460) -> (array=w1459:u32[])
                n440 = Index Array(array=w1459, index=0) -> (element=→"GB sit":u32)
                n441 = Replace Array Subset(array=w1475, new element=w1473, index=0) -> (w1471:cluster{u32, u32}[])
                n442 = property class="Bool"(reference=w1472, error in=w1456, "Colors [4]"=w1471) -> (error out=w1469:errorcluster)  [unwired: 1 out]
                n443 = Replace Array Subset(array=w1455, new element=w1452, index (row)=w1451, index (col)=7 ("disabled index (col)")) -> (w1454:dbl[][])
                n444 = Increment(x=w1451) -> (x+1=w1462:i32)
                n445 = property class="Bool"(reference=w1470, error in=w1469) -> (reference out=w1465:refnum<vi>, error out=w1464:errorcluster, "Colors [4]"=w1467:cluster{u32, u32}[])
                n446 = Replace Array Subset(array=w1467, new element=w1466, index=0) -> (w1463:cluster{u32, u32}[])
                n447 = property class="Bool"(reference=w1465, error in=w1464, "Colors [4]"=w1463) -> (error out=w1461:errorcluster)  [unwired: 1 out]
              }
              frame #9 {
                # "write in database"
                n448 = property on="Sync" class="Bool (strict)"(error in=w1495) -> (error out=w1491:errorcluster, "Value"=w1493:bool)  [unwired: 1 in, 1 out]
                n449 = property on="Frm False" class="Bool (strict)"(error in=w1491) -> (error out=w1490:errorcluster, "Value"=w1494:bool)  [unwired: 1 in, 1 out]
                n450 = Not(x=w1494) -> (.not. x?=w1492:bool)
                n451 = And(x=w1493, y=w1492) -> (x .and. y?=w1485:bool)
                n452 = call "pallet DB 2.vi"("pallet_num"=w1489, "info array"=w1496, "set data"=w1485, "error in"=w1490) -> ("error out"=w1486:errorcluster)  [unwired: 23 in]
              }
              frame #10 {
                n453 = call "defects database.vi"("Array 2"=w1508, "table"="defect_table", "pallet number"=w1507, "curv number"=w1506, "error in (no error)"=w1504, "condition"=w1502) -> ("error out"=w1505:errorcluster)  [unwired: 13 in]
              }
              frame #11 {
                n454 = property on="capture or not? 2" class="Bool (strict)"("Value"=FALSE ("capture or not? 2")) -> ()  [unwired: 2 in, 2 out]
              }
            }
          }
        }
      }
      event "Refresh Button": Mouse Down {
        # "syncron rotate"
        n455 = event-data() -> ()  [unwired: 1 in, 8 out]
        n456 = In Range and Coerce(upper limit=i16 232, x="PLT NUM SYNC", lower limit=i16 1) -> (In Range?=w1525:bool)  [unwired: 1 out]
        n457 = case shown="True" w1525 {
          selector: w1525 -> [w1543 _]
          tunnel: w1536 -> [w1540 w1570]
          tunnel: w1535 -> [w1539 w1569]
          tunnel: [w1540 w1554] -> w1534
          tunnel: [w1539 w1565] -> w1533
          tunnel: w1529 -> [w1541 w1561]
          tunnel: [w1541 w1560] -> w1528
          tunnel: "PLT NUM SYNC" -> [_ w1557]
          tunnel: w1524 -> [w1538 w1556]
          tunnel: [w1537 w1555] -> w1523
          frame False {
            n458 = Not(x=w1543) -> (.not. x?=w1542:bool)
            n459 = call "Display Message to User"("error in (no error)"=w1538, "Enable"=w1542) -> ("error out"=w1537:errorcluster)  [unwired: 8 in, 1 out]
          }
          frame True {
            w1549 = 232 ("y")
            n460 = control-ref of="232"() -> (w1568:refnum<vi>)
            n461 = property class="Bool"(reference=w1568, error in=w1556) -> (error out=w1555:errorcluster, "BoolText.Text"=w1567:string)  [unwired: 1 out]
            n462 = Decimal String To Number(string=w1567) -> (number=w1566:i32)  [unwired: 2 in, 1 out]
            n463 = Subtract(x=w1557, y=w1566) -> (x-y=w1562:i32)
            n464 = for {
              tunnel: w1570 -> [w1592] mode=indexing
              tunnel: w1569 -> [w1591] mode=indexing
              tunnel: [w1590] -> w1571 mode=indexing
              tunnel: [w1589] -> w1564 mode=indexing
              tunnel: [w1588] -> w1563 mode=indexing
              n465 = property class="Bool"(reference=w1592, error in=w1591) -> (reference out=w1589:refnum<vi>, error out=w1588:errorcluster, "BoolText.Text"=w1590:string)
            }
            n466 = Rotate 1D Array(1:w1571, 2:w1562) -> (0:w1572:string[])
            n467 = for {
              tunnel: w1572 -> [w1587] mode=indexing
              tunnel: [w1586] -> w1554 mode=indexing
              tunnel: [w1585] -> w1565 mode=indexing
              tunnel: w1564 -> [w1584] mode=indexing
              tunnel: w1563 -> [w1583] mode=indexing
              n468 = property class="Bool"(reference=w1584, error in=w1583, "BoolText.Text"=w1587) -> (reference out=w1586:refnum<vi>, error out=w1585:errorcluster)
            }
            n469 = Index Array(array=w1554, index=0) -> (element=w1552:refnum<vi>)
            n470 = for {
              N: 15 -> [_]
              tunnel: w1562 -> [w1579]
              shift-right: [w1574] -> w1560
              shift-left: w1561 -> [w1575]
              i -> [w1573]
              n471 = Array Subset(array=w1575, index (row)=0 ("index"), index (col)=w1573, length (col)=1 ("length")) -> (w1577:dbl[][])  [unwired: 1 in]
              n472 = Reshape Array(w1577, 232 ("dimension size")) -> (w1580:dbl[])
              n473 = Rotate 1D Array(1:w1580, 2:w1579) -> (0:w1576:dbl[])
              n474 = Replace Array Subset(array=w1575, new element=w1576, index (col)=w1573) -> (w1574:dbl[][])  [unwired: 1 in]
            }
            n475 = property class="Bool"(reference=w1552) -> ("BoolText.Text"=w1545:string)  [unwired: 1 in, 2 out]
            n476 = property on="PLT NUM :" class="Str"("Value"=w1545) -> ()  [unwired: 2 in, 2 out]
            n477 = Decimal String To Number(string=w1545) -> (number=w1550:i32)  [unwired: 2 in, 1 out]
            n478 = Add(x=w1550, y=45) -> (x+y=w1546:i32)
            n479 = Greater?(x=w1546, y=w1549) -> (0:w1548:bool)
            n480 = Subtract(x=w1546, y=w1549) -> (x-y=w1547:i32)
            n481 = Select(t=w1547, s=w1548, f=w1546) -> (s? t:f=w1544:i32)
            n482 = property on="Sen Plt\nNUM" class="DigNum (strict)"("Value"=w1544) -> ()  [unwired: 2 in, 2 out]
            "Sync" <- TRUE ("Sync")
          }
        }
      }
    }
    "error out" <- w1009
    "Array" <- w1010
    n483 = Wait (ms)(milliseconds to wait=u32 10) -> ()  [unwired: 1 out]
    n484 = shared-variable ".\\setting Lib.lvlib\\StopOk"() -> (w1008:bool)  [unwired: 1 in, 1 out]
  }
  "main loop stop" <- w34
  "Array 2" <- w21
  n485 = while {
    tunnel: w60 -> [w1595]
    tunnel: w42 -> [w1594]
    tunnel: [w1593] -> w35
    stop <- w1593 stop-if-true
    n486 = event shown="[5] \"capture\": Mouse Down" {
      selector: _ -> [_ _ _ _ _ _ _ _ _ _]
      dyn-events: _ -> [_ _ _ _ _ _ _ _ _ _]
      timeout: 0 -> [_ _ _ _ _ _ _ _ _ _]
      tunnel: w1595 -> [_ _ _ _ w1648 _ _ _ _ _]
      tunnel: [w1598 w1602 _ _ w1646 _ w1680 _ w1685 _] -> _
      tunnel: w1594 -> [w1598 w1604 _ _ w1647 _ _ _ w1686 _]
      tunnel: [_ _ _ _ _ _ _ _ _ w1688] -> w1593
      event Timeout {
        n487 = event-data() -> ()  [unwired: 1 in, 3 out]
        n488 = shared-variable ".\\setting Lib.lvlib\\userFlag"() -> (w1599:bool)  [unwired: 1 in, 1 out]
        n489 = case shown="True" w1599 {
          frame False {
          }
          frame True {
            n490 = property on="Login" class="Bool (strict)"("Value"=FALSE ("Login")) -> ()  [unwired: 2 in, 2 out]
            n491 = property on="setting" class="Bool"("DisabledEnum"=T4."Enabled" ("Disabled")) -> ()  [unwired: 2 in, 2 out]
          }
        }
      }
      event "Login": Mouse Down {
        n492 = event-data() -> ("CtlRef"=w1606:refnum<vi>)  [unwired: 1 in, 7 out]
        n493 = property class="Bool (strict)"(reference=w1606, error in=w1604) -> (error out=w1603:errorcluster, "Value"=w1605:bool)  [unwired: 1 out]
        n494 = case shown="False" w1605 {
          tunnel: w1603 -> [w1609 w1612]
          tunnel: [w1608 w1611] -> w1602
          frame False {
            n495 = shared-variable ".\\setting Lib.lvlib\\userFlag"(FALSE ("userFlag"), error in=w1609) -> (error out=w1608:errorcluster)
            n496 = property on="setting" class="Bool"("DisabledEnum"=T4."Disabled and Grayed Out" ("Disabled")) -> ()  [unwired: 2 in, 2 out]
          }
          frame True {
            n497 = flat-sequence {
              tunnel: [w1615] -> w1613
              tunnel: w1612 -> [w1614]
              tunnel: w1613 -> [w1622]
              tunnel: [w1621] -> w1611
              frame #0 {
                n498 = shared-variable ".\\setting Lib.lvlib\\userTisVI"() -> (w1619:refnum<vi>)  [unwired: 1 in, 1 out]
                n499 = invoke class="VI" method="FP.Open"(reference=w1619, error in=w1614, "Activate"=TRUE ("Activate?"), "State"=T13."Standard") -> (reference out=w1616:refnum<vi>, error out=w1615:errorcluster)  [unwired: 1 in, 3 out]
                n500 = shared-variable ".\\setting Lib.lvlib\\userTisVI"(w1616) -> ()  [unwired: 1 in, 1 out]
              }
              frame #1 {
                n501 = shared-variable ".\\setting Lib.lvlib\\focus"(error in=w1622) -> (w1624:refnum<vi>, error out=w1623:errorcluster)
                n502 = property class="Str"(reference=w1624, error in=w1623, "Key Focus"=TRUE) -> (error out=w1621:errorcluster)  [unwired: 1 out]
              }
            }
          }
        }
      }
      event "setting": Mouse Down {
        n503 = event-data() -> ("CtlRef"=w1626:refnum<vi>)  [unwired: 1 in, 7 out]
        n504 = property class="Bool"(reference=w1626) -> ("DisabledEnum"=w1625:T4)  [unwired: 1 in, 2 out]
        n505 = case shown="\"Enabled\"" w1625 {
          frame "Enabled" {
            n506 = shared-variable ".\\setting Lib.lvlib\\SettingThisVI"() -> (w1629:refnum<vi>)  [unwired: 1 in, 1 out]
            n507 = invoke class="VI" method="FP.Open"(reference=w1629, "Activate"=FALSE ("Activate?"), "State"=T13."Standard") -> ()  [unwired: 2 in, 5 out]
          }
          frame "Disabled", Default {
          }
        }
      }
      event "Graph Button": Mouse Down {
        n508 = event-data() -> ()  [unwired: 1 in, 8 out]
        n509 = shared-variable ".\\Waveforms.lvlib\\WaveFormThisVI"() -> (w1632:refnum<vi>)  [unwired: 1 in, 1 out]
        n510 = invoke class="VI" method="FP.Open"(reference=w1632, "Activate"=TRUE ("Activate?"), "State"=T13."Standard") -> ()  [unwired: 2 in, 5 out]
      }
      event "232", "231", "230", "229", "228", "227", "226", "225", "224", "223", "222", "221", "220", "219", "218", "217", "216", "215", "214", "213", "212", "211", "210", "209", "208", "207", "206", "205", "204", "203", "202", "201", "200", "199", "198", "197", "196", "195", "194", "193", "192", "191", "190", "189", "188", "187", "186", "185", "184", "183", "182", "181", "180", "179", "178", "177", "176", "175", "174", "173", "172", "171", "170", "169", "168", "167", "166", "165", "164", "163", "162", "161", "160", "159", "158", "157", "156", "155", "154", "153", "152", "151", "150", "149", "148", "147", "146", "145", "144", "143", "142", "141", "140", "139", "138", "137", "136", "135", "134", "133", "132", "131", "130", "129", "128", "127", "126", "125", "124", "123", "122", "121", "120", "119", "118", "117", "116", "115", "114", "113", "112", "111", "110", "109", "108", "107", "106", "105", "104", "103", "102", "101", "100", "99", "98", "97", "96", "95", "94", "93", "92", "91", "90", "89", "88", "87", "86", "85", "84", "83", "82", "81", "80", "79", "78", "77", "76", "75", "74", "73", "72", "71", "70", "69", "68", "67", "66", "65", "64", "63", "62", "61", "60", "59", "58", "57", "56", "55", "54", "53", "52", "51", "50", "49", "48", "47", "46", "45", "44", "43", "42", "41", "40", "39", "38", "37", "36", "35", "34", "33", "32", "31", "30", "29", "28", "27", "26", "25", "24", "23", "22", "21", "20", "19", "18", "17", "16", "15", "14", "13", "12", "11", "10", "9", "8", "7", "6", "5", "4", "3", "2", "1": Mouse Down {
        n511 = event-data() -> ("CtlRef"=w1649:refnum<vi>)  [unwired: 1 in, 7 out]
        n512 = shared-variable ".\\setting Lib.lvlib\\General Setting"() -> (w1645:T6)  [unwired: 1 in, 1 out]
        n513 = Unbundle By Name(w1645) -> ("Img Path"=w1644:path)
        n514 = flat-sequence {
          tunnel: [w1659] -> w1643
          tunnel: w1647 -> [w1655]
          tunnel: w1644 -> [w1651]
          tunnel: w1648 -> [w1650]
          tunnel: w1649 -> [w1658]
          tunnel: [w1654] -> w1642
          tunnel: [w1653] -> w1641
          tunnel: [w1652] -> w1639
          tunnel: [w1651] -> w1637
          tunnel: [w1650] -> w1635
          tunnel: w1643 -> [w1660]
          tunnel: w1642 -> [w1666]
          tunnel: w1641 -> [w1665]
          tunnel: [w1665] -> w1640
          tunnel: w1639 -> [w1664]
          tunnel: [w1664] -> w1638
          tunnel: w1637 -> [w1663]
          tunnel: [w1663] -> w1636
          tunnel: w1635 -> [w1662]
          tunnel: [w1662] -> w1634
          tunnel: [w1661] -> w1633
          tunnel: [w1669] -> w1646
          tunnel: w1640 -> [w1674]
          tunnel: w1638 -> [w1673]
          tunnel: w1636 -> [w1672]
          tunnel: w1634 -> [w1671]
          tunnel: w1633 -> [w1670]
          frame #0 {
            n515 = property class="Bool"(reference=w1658, error in=w1655) -> (error out=w1656:errorcluster, "BoolText.Text"=w1657:string)  [unwired: 1 out]
            n516 = property on="Array" class="Arr (strict)"() -> ("Value"=w1653:dbl[][])  [unwired: 2 in, 2 out]
            n517 = Decimal String To Number(string=w1657) -> (number=w1652:i32)  [unwired: 2 in, 1 out]
            n518 = call "pallet show.vi"("Array"=w1653, "palet num"=w1652, "File Path"=w1651, "Image 2"=w1650, "error in (no error)"=w1656) -> ("This VI"=w1654:refnum<vi>, "error out"=w1659:errorcluster)  [unwired: 13 in]
          }
          frame #1 {
            n519 = invoke class="VI" method="FP.Open"(reference=w1666, error in=w1660, "Activate"=TRUE ("Activate?"), "State"=T13."Standard") -> (error out=w1661:errorcluster)  [unwired: 1 in, 4 out]
          }
          frame #2 {
            n520 = call "pallet show.vi"("Array"=w1674, "palet num"=w1673, "File Path"=w1672, "Image 2"=w1671, "error in (no error)"=w1670) -> ("error out"=w1669:errorcluster)  [unwired: 13 in, 1 out]
          }
        }
      }
      event "capture": Mouse Down {
        n521 = event-data() -> ()  [unwired: 1 in, 8 out]
        n522 = property on="Col. Count" class="Bool (strict)"() -> ("Value"=w1676:bool)  [unwired: 2 in, 2 out]
        n523 = Not(x=w1676) -> (.not. x?=w1675:bool)
        n524 = case shown="True" w1675 {
          frame False {
          }
          frame True {
            n525 = property on="Sync" class="Bool (strict)"("Value"=FALSE ("Sync")) -> ()  [unwired: 2 in, 2 out]
            "capture or not?" <- TRUE ("capture or not?")
            "capture or not? 2" <- TRUE ("capture or not? 2")
          }
        }
      }
      event "report": Mouse Down {
        n526 = event-data() -> ()  [unwired: 1 in, 8 out]
        n527 = shared-variable ".\\setting Lib.lvlib\\QueryThisVI"() -> (w1683:refnum<vi>)  [unwired: 1 in, 1 out]
        n528 = invoke class="VI" method="FP.Open"(reference=w1683, "Activate"=TRUE ("Activate?"), "State"=T13."Standard") -> (error out=w1680:errorcluster)  [unwired: 2 in, 4 out]
      }
      event "OFF": Mouse Down {
        w1684 = FALSE ("Blinking")
        n529 = event-data() -> ()  [unwired: 1 in, 8 out]
        n530 = property on="Alarm" class="Bool (strict)"("Blinking"=w1684) -> ()  [unwired: 2 in, 2 out]
        n531 = property on="Alarm" class="Bool (strict)"("Value"=w1684) -> ()  [unwired: 2 in, 2 out]
      }
      event "Sequence Button": Mouse Down {
        n532 = event-data() -> ()  [unwired: 1 in, 8 out]
        n533 = shared-variable ".\\setting Lib.lvlib\\DefectsDatabaseThisVI"() -> (w1687:refnum<vi>)  [unwired: 1 in, 1 out]
        n534 = invoke class="VI" method="FP.Open"(reference=w1687, error in=w1686) -> (error out=w1685:errorcluster)  [unwired: 3 in, 4 out]
      }
      event "stop 3": Mouse Down {
        n535 = event-data() -> ()  [unwired: 1 in, 8 out]
        n536 = call "close.vi"("Enable"="stop 3") -> ("YES"=w1688:bool)  [unwired: 17 in, 1 out]
        "stop ok" <- w1688
        n537 = shared-variable ".\\setting Lib.lvlib\\StopOk"(w1688) -> ()  [unwired: 1 in, 1 out]
      }
    }
    n538 = Wait (ms)(milliseconds to wait=u32 10) -> ()  [unwired: 1 out]
  }
  "event loop stop" <- w35
  n539 = call "IMAQ Dispose"("All Images? (No)"=TRUE, "Image"=w51, "error in (no error)"=w48) -> ("error out"=→"camera error out":errorcluster)  [unwired: 3 in]
  n540 = property on="GB sit" class="ColBox"("Value"=u32 16448250 ("GB sit")) -> ()  [unwired: 2 in, 2 out]
  n541 = TCP Close Connection(connection ID=w38, error in (no error)=w37) -> (error out=→"error out 5":errorcluster)  [unwired: 1 in, 1 out]
  n542 = Close Python Session(session in=w71, error in=w58) -> (11:→"error out 3":errorcluster)
  n543 = while {
    stop <- FALSE stop-if-true
    n544 = property on="event loop stop" class="Bool (strict)"() -> ("Value"=w1694:bool)  [unwired: 2 in, 2 out]
    n545 = property on="stop live view" class="Bool (strict)"() -> ("Value"=w1690:bool)  [unwired: 2 in, 2 out]
    n546 = property on="sensor loop stop" class="Bool (strict)"() -> ("Value"=w1695:bool)  [unwired: 2 in, 2 out]
    n547 = property on="main loop stop" class="Bool (strict)"() -> ("Value"=w1691:bool)  [unwired: 2 in, 2 out]
    n548 = Compound Arithmetic op=AND(w1691, w1690, w1695, w1694) -> (w1696:bool)
    n549 = Quit LabVIEW(quit? (T)=w1696) -> ()
    n550 = Wait (ms)(milliseconds to wait=u32 10) -> ()  [unwired: 1 out]
  }
  "Alarm" <- FALSE ("Alarm")
